vi "DblMonoPMDCurrentScan.vi"() -> ()   [LabVIEW 2010]
uses:
  <vilib>/DAQmx/write.llb/DAQmx Write (Analog DBL 1Chan 1Samp).vi
  <vilib>/DAQmx/read.llb/DAQmx Read (Analog 1D DBL 1Chan NSamp).vi
  <vilib>/DAQmx/create/channels.llb/DAQmx Create Channel (AO-Voltage-Basic).vi
  <vilib>/DAQmx/create/channels.llb/DAQmx Create Channel (AI-Voltage-Basic).vi
  <vilib>/daqmx/miscellaneous.llb/DAQmx Fill In Error Info.vi
  <vilib>/DAQmx/configure/timing.llb/DAQmx Timing (Sample Clock).vi
  <vilib>/Utility/file.llb/Write To Spreadsheet File (DBL).vi
  <vilib>/Analysis/NI_AALBase.lvlib
panel:
  in  "Voltage B":dbl min=-10.0 max=10.0 step=0.1 format="%0.2f"
  in  "Voltage A":dbl min=-10.0 max=10.0 step=0.1 format="%0.2f"
  in  "Output B":tag="Dev1/ao3"
  in  "Output A":tag="Dev1/ao2"
  in  "Input Channel":tag="Dev1/ai6"
  in  "Current":bool
  in  "Power":bool=TRUE
  out "ScanGraph":cluster{dbl[], dbl[]}(graph)
  in  "Sensitivity":dbl=1e-09 caption="(A/V)" format="%#_6p"
  out "Readout":dbl=-2.45576047e-07 format="%^#_9e"
  in  "Scan Save Path":path
  in  "On":bool=TRUE
  out "Waveform Chart":dbl(graph)=-2.45576047e-07
  in  "Save":bool=TRUE
  in  "Exit":bool
  in  "STOP":bool
  in  "Step Time (sec)":dbl=1.0 min=0.001 max=300.0 step=0.001 format="%.3f"
  in  "Step Size (nm)":dbl=1.0 min=0.1 max=100.0 step=0.1 format="%.1f"
  in  "End":dbl=800.0 min=0.0 max=2000.0 step=0.1 format="%.1f"
  in  "Start":dbl=400.0 min=0.0 max=2000.0 step=0.1 format="%.1f"
  in  "Scan":bool
  in  "Up":bool=TRUE caption="Down"
  in  "Increment (nm)":dbl=10.0 min=0.1 max=2000.0 step=0.1 format="%.1f"
  in  "PMD Settings":T1={"Beam Diameter (mm)"=4.0, "BWIn"=0, "Averaging Rate"=300, "Auto Range"=TRUE} {"Averaging Rate" min=33 max=5000 step=1; "BWIn" items=["HIGH", "LOW"]; "Beam Diameter (mm)" min=1.0 max=9.0 step=0.5}
  in  "Step":bool
  out "Busy":bool=TRUE
  in  "Send Command":bool
  in  "Command":u16(ring)=1 items=["nm", "goto", "nm/min", "VIS grating", "IR grating"]
  in  "Wavelength (nm)":dbl=500.0 min=0.0 max=2000.0 step=0.1 format="%.1f"
  in  "Scan Speed (nm/min)":dbl=100.0 min=1.0 max=500.0 step=0.1 format="%.1f"
  out "Done?":string="   ..."
  in  "Send Question":bool
  in  "Ask?":u16(ring) items=["?nm", "?nm/min", "?grating", "?turret", "?gratings"]
  in  "Zero?":bool
  out "PM Error log":string="-222,\"Data out of range\"\n-222,\"Data out of range\"\n-222,\"Data out of range\"\n-222,\"Data out of range\"\n-222,\"Data out of range\"\n-222,\"Data out of range\"\n-222,\"Data out of range\"\n-222,\"Data out of range\"\n-222,\"Data out of range\"\n-222,\"Data out of range\"\n-222,\"Data out of range\"\n-222,\"Data out of range\"\n-222,\"Data out of range\"\n-222,\"Data out of range\"\n-222,\"Data out of range\"\n-222,\"Data out of range\"\n-222,\"Data out of range\"\n-222,\"Data out of range\"\n-222,\"Data out of range\"\n-222,\"Data out of range\"\n-222,\"Data out of range\"\n-222,\"Data out of range\"\n-222,\"Data out of range\"\n-222,\"Data out of range\"\n-222,\"Data out of range\"\n-222,\"Data out of range\"\n-222,\"Data out of range\"\n-222,\"Data out of range\"\n-222,\"Data out of range\"\n-222,\"Data out of range\"\n-222,\"Data out of range\"\n-222,\"Data out of range\"\n-222,\"Data out of range\"\n-222,\"Data out of range\"\n-222,\"Data out of range\"\n-222,\"Data out of range\"\n-222,\"Data out of range\"\n-222,\"Data out of range\"\n-222,\"Data out of range\"\n-222,\"Data out of range\"\n-222,\"Data out of range\"\n-222,\"Data out of range\"\n-222,\"Data out of range\"\n-222,\"Data out of range\"\n-222,\"Data out of range\"\n-222,\"Data out of range\"\n-222,\"Data out of range\"\n-222,\"Data out of range\"\n-222,\"Data out of range\"\n-222,\"Data out of range\"\n-222,\"Data out of range\"\n-222,\"Data out of range\"\n-222,\"Data out of range\"\n-222,\"Data out of range\"\n-222,\"Data out of range\"\n-222,\"Data out of range\"\n-222,\"Data out of range\"\n-222,\"Data out of range\"\n-222,\"Data out of range\"\n-222,\"Data out of range\"\n-222,\"Data out of range\"\n-222,\"Data out of range\"\n-222,\"Data out of range\"\n-222,\"Data out of range\"\n-222,\"Data out of range\"\n-222,\"Data out of range\"\n-222,\"Data out of range\"\n-222,\"Data out of range\"\n-222,\"Data out of range\"\n-222,\"Data out of range\"\n-222,\"Data out of range\"\n-222,\"Data out of range\"\n-222,\"Data out of range\"\n-222,\"Data out of range\"\n-222,\"Data out of range\"\n-222,\"Data out of range\"\n-222,\"Data out of range\"\n-222,\"Data out of range\"\n-222,\"Data out of range\"\n-222,\"Data out of range\"\n-222,\"Data out of range\"\n-222,\"Data out of range\"\n-222,\"Data out of range\"\n-222,\"Data out of range\"\n-222,\"Data out of range\"\n-222,\"Data out of range\"\n-222,\"Data out of range\"\n-222,\"Data out of range\"\n-222,\"Data out of range\"\n-222,\"Data out of range\"\n-222,\"Data out of range\"\n-222,\"Data out of range\"\n-222,\"Data out of range\"\n-222,\"Data out of range\"\n-222,\"Data out of range\"\n-222,\"Data out of range\"\n-222,\"Data out of range\"\n-222,\"Data out of range\"\n-222,\"Data out of range\"\n-222,\"Data out of range\"\n-222,\"Data out of range\"\n-222,\"Data out of range\"\n-222,\"Data out of range\"\n-222,\"Data out of range\"\n-222,\"Data out of range\"\n-222,\"Data out of range\"\n-222,\"Data out of range\"\n-222,\"Data out of range\"\n-222,\"Data out of range\"\n-222,\"Data out of range\"\n-222,\"Data out of range\"\n-222,\"Data out of range\"\n-222,\"Data out of range\"\n-222,\"Data out of range\"\n-222,\"Data out of range\"\n-222,\"Data out of range\"\n-222,\"Data out of range\"\n-222,\"Data out of range\"\n-222,\"Data out of range\"\n-222,\"Data out of range\"\n-222,\"Data out of range\"\n-222,\"Data out of range\"\n-222,\"Data out of range\"\n-222,\"Data out of range\"\n-222,\"Data out of range\"\n-222,\"Data out of range\"\n-222,\"Data out of range\"\n-222,\"Data out of range\"\n-222,\"Data out of range\"\n-222,\"Data out of range\"\n-222,\"Data out of range\"\n-222,\"Data out of range\"\n-222,\"Data out of range\"\n-222,\"Data out of range\"\n-222,\"Data out of range\"\n-222,\"Data out of range\"\n-222,\"Data out of range\"\n-222,\"Data out of range\"\n-222,\"Data out of range\"\n-222,\"Data out of range\"\n-222,\"Data out of range\"\n-222,\"Data out of range\"\n-222,\"Data out of range\"\n-222,\"Data out of range\"\n-222,\"Data out of range\"\n-222,\"Data out of range\"\n-222,\"Data out of range\"\n-222,\"Data out of range\"\n-222,\"Data out of range\"\n-222,\"Data out of range\"\n-222,\"Data out of range\"\n-222,\"Data out of range\"\n-222,\"Data out of range\"\n-222,\"Data out of range\"\n-222,\"Data out of range\"\n-222,\"Data out of range\"\n-222,\"Data out of range\"\n-222,\"Data out of range\"\n-222,\"Data out of range\"\n-222,\"Data out of range\"\n-222,\"Data out of range\"\n-222,\"Data out of range\"\n-222,\"Data out of range\"\n-222,\"Data out of range\"\n-222,\"Data out of range\"\n-222,\"Data out of range\"\n-222,\"Data out of range\"\n-222,\"Data out of range\"\n-222,\"Data out of range\"\n-222,\"Data out of range\"\n-222,\"Data out of range\"\n-222,\"Data out of range\"\n-222,\"Data out of range\"\n-222,\"Data out of range\"\n-222,\"Data out of range\"\n-222,\"Data out of range\"\n-222,\"Data out of range\"\n-222,\"Data out of range\"\n-222,\"Data out of range\"\n-222,\"Data out of range\"\n-222,\"Data out of range\"\n-222,\"Data out of range\"\n-222,\"Data out of range\"\n-222,\"Data out of range\"\n-222,\"Data out of range\"\n-222,\"Data out of range\"\n-222,\"Data out of range\"\n-222,\"Data out of range\"\n-222,\"Data out of range\"\n-222,\"Data out of range\"\n-222,\"Data out of range\"\n-222,\"Data out of range\"\n-222,\"Data out of range\"\n-222,\"Data out of range\"\n-222,\"Data out of range\"\n-222,\"Data out of range\"\n-222,\"Data out of range\"\n-222,\"Data out of range\"\n-222,\"Data out of range\"\n-222,\"Data out of range\"\n-222,\"Data out of range\"\n-222,\"Data out of range\"\n-222,\"Data out of range\"\n-222,\"Data out of range\"\n-222,\"Data out of range\"\n-222,\"Data out of range\"\n-222,\"Data out of range\"\n-222,\"Data out of range\"\n-222,\"Data out of range\"\n-222,\"Data out of range\"\n-222,\"Data out of range\"\n-222,\"Data out of range\"\n-222,\"Data out of range\"\n-222,\"Data out of range\"\n-222,\"Data out of range\"\n-222,\"Data out of range\"\n-222,\"Data out of range\"\n-222,\"Data out of range\"\n-222,\"Data out of range\"\n-222,\"Data out of range\"\n-222,\"Data out of range\"\n-222,\"Data out of range\"\n-222,\"Data out of range\"\n-222,\"Data out of range\"\n-222,\"Data out of range\"\n-222,\"Data out of range\"\n-222,\"Data out of range\"\n-222,\"Data out of range\"\n-222,\"Data out of range\"\n-222,\"Data out of range\"\n-222,\"Data out of range\"\n-222,\"Data out of range\"\n-222,\"Data out of range\"\n-222,\"Data out of range\"\n-222,\"Data out of range\"\n-222,\"Data out of range\"\n-222,\"Data out of range\"\n-222,\"Data out of range\"\n-222,\"Data out of range\"\n-222,\"Data out of range\"\n-222,\"Data out of range\"\n-222,\"Data out of range\"\n-222,\"Data out of range\"\n-222,\"Data out of range\"\n-222,\"Data out of range\"\n-222,\"Data out of range\"\n-222,\"Data out of range\"\n-222,\"Data out of range\"\n-222,\"Data out of range\"\n-222,\"Data out of range\"\n-222,\"Data out of range\"\n-222,\"Data out of range\"\n-222,\"Data out of range\"\n-222,\"Data out of range\"\n-222,\"Data out of range\"\n-222,\"Data out of range\"\n-222,\"Data out of range\"\n-222,\"Data out of range\"\n-222,\"Data out of range\"\n-222,\"Data out of range\"\n-222,\"Data out of range\"\n-222,\"Data out of range\"\n-222,\"Data out of range\"\n-222,\"Data out of range\"\n-222,\"Data out of range\"\n-222,\"Data out of range\"\n-222,\"Data out of range\"\n-222,\"Data out of range\"\n-222,\"Data out of range\"\n-222,\"Data out of range\"\n-222,\"Data out of range\"\n-222,\"Data out of range\"\n-222,\"Data out of range\"\n-222,\"Data out of range\"\n-222,\"Data out of range\"\n-222,\"Data out of range\"\n-222,\"Data out of range\"\n-222,\"Data out of range\"\n-222,\"Data out of range\"\n-222,\"Data out of range\"\n-222,\"Data out of range\"\n-222,\"Data out of range\"\n-222,\"Data out of range\"\n-222,\"Data out of range\"\n-222,\"Data out of range\"\n-222,\"Data out of range\"\n-222,\"Data out of range\"\n-222,\"Data out of range\"\n-222,\"Data out of range\"\n-222,\"Data out of range\"\n-222,\"Data out of range\"\n-222,\"Data out of range\"\n-222,\"Data out of range\"\n-222,\"Data out of range\"\n-222,\"Data out of range\"\n-222,\"Data out of range\"\n-222,\"Data out of range\"\n-222,\"Data out of range\"\n-222,\"Data out of range\"\n-222,\"Data out of range\"\n-222,\"Data out of range\"\n-222,\"Data out of range\"\n-222,\"Data out of range\"\n-222,\"Data out of range\"\n-222,\"Data out of range\"\n-222,\"Data out of range\"\n-222,\"Data out of range\"\n-222,\"Data out of range\"\n-222,\"Data out of range\"\n-222,\"Data out of range\"\n-222,\"Data out of range\"\n-222,\"Data out of range\"\n-222,\"Data out of range\"\n-222,\"Data out of range\"\n-222,\"Data out of range\"\n-222,\"Data out of range\"\n-222,\"Data out of range\"\n-222,\"Data out of range\"\n-222,\"Data out of range\"\n-222,\"Data out of range\"\n-222,\"Data out of range\"\n-222,\"Data out of range\"\n-222,\"Data out of range\"\n-222,\"Data out of range\"\n-222,\"Data out of range\"\n-222,\"Data out of range\"\n-222,\"Data out of range\"\n-222,\"Data out of range\"\n-222,\"Data out of range\"\n-222,\"Data out of range\"\n-222,\"Data out of range\"\n-222,\"Data out of range\"\n-222,\"Data out of range\"\n-222,\"Data out of range\"\n-222,\"Data out of range\"\n-222,\"Data out of range\"\n-222,\"Data out of range\"\n-222,\"Data out of range\"\n-222,\"Data out of range\"\n-222,\"Data out of range\"\n-222,\"Data out of range\"\n-222,\"Data out of range\"\n-222,\"Data out of range\"\n-222,\"Data out of range\"\n-222,\"Data out of range\"\n-222,\"Data out of range\"\n-222,\"Data out of range\"\n-222,\"Data out of range\"\n-222,\"Data out of range\"\n-222,\"Data out of range\"\n-222,\"Data out of range\"\n-222,\"Data out of range\"\n-222,\"Data out of range\"\n-222,\"Data out of range\"\n-222,\"Data out of range\"\n-222,\"Data out of range\"\n-222,\"Data out of range\"\n-222,\"Data out of range\"\n-222,\"Data out of range\"\n-222,\"Data out of range\"\n-222,\"Data out of range\"\n-222,\"Data out of range\"\n-222,\"Data out of range\"\n-222,\"Data out of range\"\n-222,\"Data out of range\"\n-222,\"Data out of range\"\n-222,\"Data out of range\"\n-222,\"Data out of range\"\n-222,\"Data out of range\"\n-222,\"Data out of range\"\n-222,\"Data out of range\"\n-222,\"Data out of range\"\n-222,\"Data out of range\"\n-222,\"Data out of range\"\n-222,\"Data out of range\"\n-222,\"Data out of range\"\n-222,\"Data out of range\"\n-222,\"Data out of range\"\n-222,\"Data out of range\"\n-222,\"Data out of range\"\n-222,\"Data out of range\"\n-222,\"Data out of range\"\n-222,\"Data out of range\"\n-222,\"Data out of range\"\n-222,\"Data out of range\"\n-222,\"Data out of range\"\n-222,\"Data out of range\"\n-222,\"Data out of range\"\n-222,\"Data out of range\"\n-222,\"Data out of range\"\n-222,\"Data out of range\"\n-222,\"Data out of range\"\n-222,\"Data out of range\"\n-222,\"Data out of range\"\n-222,\"Data out of range\"\n-222,\"Data out of range\"\n-222,\"Data out of range\"\n-222,\"Data out of range\"\n-222,\"Data out of range\"\n-222,\"Data out of range\"\n-222,\"Data out of range\"\n-222,\"Data out of range\"\n-222,\"Data out of range\"\n-222,\"Data out of range\"\n-222,\"Data out of range\"\n-222,\"Data out of range\"\n-222,\"Data out of range\"\n-222,\"Data out of range\"\n-222,\"Data out of range\"\n-222,\"Data out of range\"\n-222,\"Data out of range\"\n-222,\"Data out of range\"\n-222,\"Data out of range\"\n-222,\"Data out of range\"\n-222,\"Data out of range\"\n-222,\"Data out of range\"\n-222,\"Data out of range\"\n-222,\"Data out of range\"\n-222,\"Data out of range\"\n-222,\"Data out of range\"\n-222,\"Data out of range\"\n-222,\"Data out of range\"\n-222,\"Data out of range\"\n-222,\"Data out of range\"\n-222,\"Data out of range\"\n-222,\"Data out of range\"\n-222,\"Data out of range\"\n-222,\"Data out of range\"\n-222,\"Data out of range\"\n-222,\"Data out of range\"\n-222,\"Data out of range\"\n-222,\"Data out of range\"\n-222,\"Data out of range\"\n-222,\"Data out of range\"\n-222,\"Data out of range\"\n-222,\"Data out of range\"\n-222,\"Data out of range\"\n-222,\"Data out of range\"\n-222,\"Data out of range\"\n-222,\"Data out of range\"\n-222,\"Data out of range\"\n-222,\"Data out of range\"\n-222,\"Data out of range\"\n-222,\"Data out of range\"\n-222,\"Data out of range\"\n-222,\"Data out of range\"\n-222,\"Data out of range\"\n-222,\"Data out of range\"\n-222,\"Data out of range\"\n-222,\"Data out of range\"\n-222,\"Data out of range\"\n-222,\"Data out of range\"\n-222,\"Data out of range\"\n-222,\"Data out of range\"\n-222,\"Data out of range\"\n-222,\"Data out of range\"\n-222,\"Data out of range\"\n-222,\"Data out of range\"\n-222,\"Data out of range\"\n-222,\"Data out of range\"\n-222,\"Data out of range\"\n-222,\"Data out of range\"\n-222,\"Data out of range\"\n-222,\"Data out of range\"\n-222,\"Data out of range\"\n-222,\"Data out of range\"\n-222,\"Data out of range\"\n-222,\"Data out of range\"\n-222,\"Data out of range\"\n-222,\"Data out of range\"\n-222,\"Data out of range\"\n-222,\"Data out of range\"\n-222,\"Data out of range\"\n-222,\"Data out of range\"\n-222,\"Data out of range\"\n-222,\"Data out of range\"\n-222,\"Data out of range\"\n-222,\"Data out of range\"\n-222,\"Data out of range\"\n-222,\"Data out of range\"\n-222,\"Data out of range\"\n-222,\"Data out of range\"\n-222,\"Data out of range\"\n-222,\"Data out of range\"\n-222,\"Data out of range\"\n-222,\"Data out of range\"\n-222,\"Data out of range\"\n-222,\"Data out of range\"\n-222,\"Data out of range\"\n-222,\"Data out of range\"\n-222,\"Data out of range\"\n-222,\"Data out of range\"\n-222,\"Data out of range\"\n-222,\"Data out of range\"\n-222,\"Data out of range\"\n-222,\"Data out of range\"\n-222,\"Data out of range\"\n-222,\"Data out of range\"\n-222,\"Data out of range\"\n-222,\"Data out of range\"\n-222,\"Data out of range\"\n-222,\"Data out of range\"\n-222,\"Data out of range\"\n-222,\"Data out of range\"\n-222,\"Data out of range\"\n-222,\"Data out of range\"\n-222,\"Data out of range\"\n-222,\"Data out of range\"\n-222,\"Data out of range\"\n-222,\"Data out of range\"\n-222,\"Data out of range\"\n-222,\"Data out of range\"\n-222,\"Data out of range\"\n-222,\"Data out of range\"\n-222,\"Data out of range\"\n-222,\"Data out of range\"\n-222,\"Data out of range\"\n-222,\"Data out of range\"\n-222,\"Data out of range\"\n-222,\"Data out of range\"\n-222,\"Data out of range\"\n-222,\"Data out of range\"\n-222,\"Data out of range\"\n-222,\"Data out of range\"\n-222,\"Data out of range\"\n-222,\"Data out of range\"\n-222,\"Data out of range\"\n-222,\"Data out of range\"\n-222,\"Data out of range\"\n-222,\"Data out of range\"\n-222,\"Data out of range\"\n-222,\"Data out of range\"\n-222,\"Data out of range\"\n-222,\"Data out of range\"\n-222,\"Data out of range\"\n-222,\"Data out of range\"\n-222,\"Data out of range\"\n-222,\"Data out of range\"\n-222,\"Data out of range\"\n-222,\"Data out of range\"\n-222,\"Data out of range\"\n-222,\"Data out of range\"\n-222,\"Data out of range\"\n-222,\"Data out of range\"\n-222,\"Data out of range\"\n-222,\"Data out of range\"\n-222,\"Data out of range\"\n-222,\"Data out of range\"\n-222,\"Data out of range\"\n-222,\"Data out of range\"\n-222,\"Data out of range\"\n-222,\"Data out of range\"\n-222,\"Data out of range\"\n-222,\"Data out of range\"\n-222,\"Data out of range\"\n-222,\"Data out of range\"\n-222,\"Data out of range\"\n-222,\"Data out of range\"\n-222,\"Data out of range\"\n-222,\"Data out of range\"\n-222,\"Data out of range\"\n-222,\"Data out of range\"\n-222,\"Data out of range\"\n-222,\"Data out of range\"\n-222,\"Data out of range\"\n-222,\"Data out of range\"\n-222,\"Data out of range\"\n-222,\"Data out of range\"\n-222,\"Data out of range\"\n-222,\"Data out of range\"\n-222,\"Data out of range\"\n-222,\"Data out of range\"\n-222,\"Data out of range\"\n-222,\"Data out of range\"\n-222,\"Data out of range\"\n-222,\"Data out of range\"\n-222,\"Data out of range\"\n-222,\"Data out of range\"\n-222,\"Data out of range\"\n-222,\"Data out of range\"\n-222,\"Data out of range\"\n-222,\"Data out of range\"\n-222,\"Data out of range\"\n-222,\"Data out of range\"\n-222,\"Data out of range\"\n-222,\"Data out of range\"\n-222,\"Data out of range\"\n-222,\"Data out of range\"\n-222,\"Data out of range\"\n-222,\"Data out of range\"\n-222,\"Data out of range\"\n-222,\"Data out of range\"\n-222,\"Data out of range\"\n-222,\"Data out of range\"\n-222,\"Data out of range\"\n-222,\"Data out of range\"\n-222,\"Data out of range\"\n-222,\"Data out of range\"\n-222,\"Data out of range\"\n-222,\"Data out of range\"\n-222,\"Data out of range\"\n-222,\"Data out of range\"\n-222,\"Data out of range\"\n-222,\"Data out of range\"\n-222,\"Data out of range\"\n-222,\"Data out of range\"\n-222,\"Data out of range\"\n-222,\"Data out of range\"\n-222,\"Data out of range\"\n-222,\"Data out of range\"\n-222,\"Data out of range\"\n-222,\"Data out of range\"\n-222,\"Data out of range\"\n-222,\"Data out of range\"\n-222,\"Data out of range\"\n-222,\"Data out of range\"\n-222,\"Data out of range\"\n-222,\"Data out of range\"\n-222,\"Data out of range\"\n-222,\"Data out of range\"\n-222,\"Data out of range\"\n-222,\"Data out of range\"\n-222,\"Data out of range\"\n-222,\"Data out of range\"\n-222,\"Data out of range\"\n-222,\"Data out of range\"\n-222,\"Data out of range\"\n-222,\"Data out of range\"\n-222,\"Data out of range\"\n-222,\"Data out of range\"\n-222,\"Data out of range\"\n-222,\"Data out of range\"\n-222,\"Data out of range\"\n-222,\"Data out of range\"\n-222,\"Data out of range\"\n-222,\"Data out of range\"\n-222,\"Data out of range\"\n-222,\"Data out of range\"\n-222,\"Data out of range\"\n-222,\"Data out of range\"\n-222,\"Data out of range\"\n-222,\"Data out of range\"\n-222,\"Data out of range\"\n-222,\"Data out of range\"\n-222,\"Data out of range\"\n-222,\"Data out of range\"\n-222,\"Data out of range\"\n-222,\"Data out of range\"\n-222,\"Data out of range\"\n-222,\"Data out of range\"\n-222,\"Data out of range\"\n-222,\"Data out of range\"\n-222,\"Data out of range\"\n-222,\"Data out of range\"\n-222,\"Data out of range\"\n-222,\"Data out of range\"\n-222,\"Data out of range\"\n-222,\"Data out of range\"\n-222,\"Data out of range\"\n-222,\"Data out of range\"\n-222,\"Data out of range\"\n-222,\"Data out of range\"\n-222,\"Data out of range\"\n-222,\"Data out of range\"\n-222,\"Data out of range\"\n-222,\"Data out of range\"\n-222,\"Data out of range\"\n-222,\"Data out of range\"\n-222,\"Data out of range\"\n-222,\"Data out of range\"\n-222,\"Data out of range\"\n-222,\"Data out of range\"\n-222,\"Data out of range\"\n-222,\"Data out of range\"\n-222,\"Data out of range\"\n-222,\"Data out of range\"\n-222,\"Data out of range\"\n-222,\"Data out of range\"\n-222,\"Data out of range\"\n-222,\"Data out of range\"\n-222,\"Data out of range\"\n-222,\"Data out of range\"\n-222,\"Data out of range\"\n-222,\"Data out of range\"\n-222,\"Data out of range\"\n-222,\"Data out of range\"\n-222,\"Data out of range\"\n-222,\"Data out of range\"\n-222,\"Data out of range\"\n-222,\"Data out of range\"\n-222,\"Data out of range\"\n-222,\"Data out of range\"\n-222,\"Data out of range\"\n-222,\"Data out of range\"\n-222,\"Data out of range\"\n-222,\"Data out of range\"\n-222,\"Data out of range\"\n-222,\"Data out of range\"\n-222,\"Data out of range\"\n-222,\"Data out of range\"\n-222,\"Data out of range\"\n-222,\"Data out of range\"\n-222,\"Data out of range\"\n-222,\"Data out of range\"\n-222,\"Data out of range\"\n-222,\"Data out of range\"\n-222,\"Data out of range\"\n-222,\"Data out of range\"\n-222,\"Data out of range\"\n-222,\"Data out of range\"\n-222,\"Data out of range\"\n-222,\"Data out of range\"\n-222,\"Data out of range\"\n-222,\"Data out of range\"\n-222,\"Data out of range\"\n-222,\"Data out of range\"\n-222,\"Data out of range\"\n-222,\"Data out of range\"\n-222,\"Data out of range\"\n-222,\"Data out of range\"\n-222,\"Data out of range\"\n-222,\"Data out of range\"\n-222,\"Data out of range\"\n-222,\"Data out of range\"\n-222,\"Data out of range\"\n-222,\"Data out of range\"\n-222,\"Data out of range\"\n-222,\"Data out of range\"\n-222,\"Data out of range\"\n-222,\"Data out of range\"\n-222,\"Data out of range\"\n-222,\"Data out of range\"\n-222,\"Data out of range\"\n-222,\"Data out of range\"\n-222,\"Data out of range\"\n-222,\"Data out of range\"\n-222,\"Data out of range\"\n-222,\"Data out of range\"\n-222,\"Data out of range\"\n-222,\"Data out of range\"\n-222,\"Data out of range\"\n-222,\"Data out of range\"\n-222,\"Data out of range\"\n-222,\"Data out of range\"\n-222,\"Data out of range\"\n-222,\"Data out of range\"\n-222,\"Data out of range\"\n-222,\"Data out of range\"\n-222,\"Data out of range\"\n-222,\"Data out of range\"\n-222,\"Data out of range\"\n-222,\"Data out of range\"\n-222,\"Data out of range\"\n-222,\"Data out of range\"\n-222,\"Data out of range\"\n-222,\"Data out of range\"\n-222,\"Data out of range\"\n-222,\"Data out of range\"\n-222,\"Data out of range\"\n-222,\"Data out of range\"\n-222,\"Data out of range\"\n-222,\"Data out of range\"\n-222,\"Data out of range\"\n-222,\"Data out of range\"\n-222,\"Data out of range\"\n-222,\"Data out of range\"\n-222,\"Data out of range\"\n-222,\"Data out of range\"\n-222,\"Data out of range\"\n-222,\"Data out of range\"\n-222,\"Data out of range\"\n-222,\"Data out of range\"\n-222,\"Data out of range\"\n-222,\"Data out of range\"\n-222,\"Data out of range\"\n-222,\"Data out of range\"\n-222,\"Data out of range\"\n-222,\"Data out of range\"\n-222,\"Data out of range\"\n-222,\"Data out of range\"\n-222,\"Data out of range\"\n-222,\"Data out of range\"\n-222,\"Data out of range\"\n-222,\"Data out of range\"\n-222,\"Data out of range\"\n-222,\"Data out of range\"\n-222,\"Data out of range\"\n-222,\"Data out of range\"\n-222,\"Data out of range\"\n-222,\"Data out of range\"\n-222,\"Data out of range\"\n-222,\"Data out of range\"\n-222,\"Data out of range\"\n-222,\"Data out of range\"\n-222,\"Data out of range\"\n-222,\"Data out of range\"\n-222,\"Data out of range\"\n-222,\"Data out of range\"\n-222,\"Data out of range\"\n-222,\"Data out of range\"\n-222,\"Data out of range\"\n-222,\"Data out of range\"\n-222,\"Data out of range\"\n-222,\"Data out of range\"\n-222,\"Data out of range\"\n-222,\"Data out of range\"\n-222,\"Data out of range\"\n-222,\"Data out of range\"\n-222,\"Data out of range\"\n-222,\"Data out of range\"\n-222,\"Data out of range\"\n-222,\"Data out of range\"\n-222,\"Data out of range\"\n-222,\"Data out of range\"\n-222,\"Data out of range\"\n-222,\"Data out of range\"\n-222,\"Data out of range\"\n-222,\"Data out of range\"\n-222,\"Data out of range\"\n-222,\"Data out of range\"\n-222,\"Data out of range\"\n-222,\"Data out of range\"\n-222,\"Data out of range\"\n-222,\"Data out of range\"\n-222,\"Data out of range\"\n-222,\"Data out of range\"\n-222,\"Data out of range\"\n-222,\"Data out of range\"\n-222,\"Data out of range\"\n-222,\"Data out of range\"\n-222,\"Data out of range\"\n-222,\"Data out of range\"\n-222,\"Data out of range\"\n-222,\"Data out of range\"\n-222,\"Data out of range\"\n-222,\"Data out of range\"\n-222,\"Data out of range\"\n-222,\"Data out of range\"\n-222,\"Data out of range\"\n-222,\"Data out of range\"\n-222,\"Data out of range\"\n-222,\"Data out of range\"\n-222,\"Data out of range\"\n-222,\"Data out of range\"\n-222,\"Data out of range\"\n-222,\"Data out of range\"\n-222,\"Data out of range\"\n-222,\"Data out of range\"\n-222,\"Data out of range\"\n-222,\"Data out of range\"\n-222,\"Data out of range\"\n-222,\"Data out of range\"\n-222,\"Data out of range\"\n-222,\"Data out of range\"\n-222,\"Data out of range\"\n-222,\"Data out of range\"\n-222,\"Data out of range\"\n-222,\"Data out of range\"\n-222,\"Data out of range\"\n-222,\"Data out of range\"\n-222,\"Data out of range\"\n-222,\"Data out of range\"\n-222,\"Data out of range\"\n-222,\"Data out of range\"\n-222,\"Data out of range\"\n-222,\"Data out of range\"\n-222,\"Data out of range\"\n-222,\"Data out of range\"\n-222,\"Data out of range\"\n-222,\"Data out of range\"\n-222,\"Data out of range\"\n-222,\"Data out of range\"\n-222,\"Data out of range\"\n-222,\"Data out of range\"\n-222,\"Data out of range\"\n-222,\"Data out of range\"\n-222,\"Data out of range\"\n-222,\"Data out of range\"\n-222,\"Data out of range\"\n-222,\"Data out of range\"\n-222,\"Data out of range\"\n-222,\"Data out of range\"\n-222,\"Data out of range\"\n-222,\"Data out of range\"\n-222,\"Data out of range\"\n-222,\"Data out of range\"\n-222,\"Data out of range\"\n-222,\"Data out of range\"\n-222,\"Data out of range\"\n-222,\"Data out of range\"\n-222,\"Data out of range\"\n-222,\"Data out of range\"\n-222,\"Data out of range\"\n-222,\"Data out of range\"\n-222,\"Data out of range\"\n-222,\"Data out of range\"\n-222,\"Data out of range\"\n-222,\"Data out of range\"\n-222,\"Data out of range\"\n-222,\"Data out of range\"\n-222,\"Data out of range\"\n-222,\"Data out of range\"\n-222,\"Data out of range\"\n-222,\"Data out of range\"\n-222,\"Data out of range\"\n-222,\"Data out of range\"\n-222,\"Data out of range\"\n-222,\"Data out of range\"\n-222,\"Data out of range\"\n-222,\"Data out of range\"\n-222,\"Data out of range\"\n-222,\"Data out of range\"\n-222,\"Data out of range\"\n-222,\"Data out of range\"\n-222,\"Data out of range\"\n-222,\"Data out of range\"\n-222,\"Data out of range\"\n-222,\"Data out of range\"\n-222,\"Data out of range\"\n-222,\"Data out of range\"\n-222,\"Data out of range\"\n-222,\"Data out of range\"\n-222,\"Data out of range\"\n-222,\"Data out of range\"\n-222,\"Data out of range\"\n-222,\"Data out of range\"\n-222,\"Data out of range\"\n-222,\"Data out of range\"\n-222,\"Data out of range\"\n-222,\"Data out of range\"\n-222,\"Data out of range\"\n-222,\"Data out of range\"\n-222,\"Data out of range\"\n-222,\"Data out of range\"\n-222,\"Data out of range\"\n-222,\"Data out of range\"\n-222,\"Data out of range\"\n-222,\"Data out of range\"\n-222,\"Data out of range\"\n-222,\"Data out of range\"\n-222,\"Data out of range\"\n-222,\"Data out of range\"\n-222,\"Data out of range\"\n-222,\"Data out of range\"\n-222,\"Data out of range\"\n-222,\"Data out of range\"\n-222,\"Data out of range\"\n-222,\"Data out of range\"\n-222,\"Data out of range\"\n-222,\"Data out of range\"\n-222,\"Data out of range\"\n-222,\"Data out of range\"\n-222,\"Data out of range\"\n-222,\"Data out of range\"\n-222,\"Data out of range\"\n-222,\"Data out of range\"\n-222,\"Data out of range\"\n-222,\"Data out of range\"\n-222,\"Data out of range\"\n-222,\"Data out of range\"\n-222,\"Data out of range\"\n-222,\"Data out of range\"\n-222,\"Data out of range\"\n-222,\"Data out of range\"\n-222,\"Data out of range\"\n-222,\"Data out of range\"\n-222,\"Data out of range\"\n-222,\"Data out of range\"\n-222,\"Data out of range\"\n-222,\"Data out of range\"\n-222,\"Data out of range\"\n-222,\"Data out of range\"\n-222,\"Data out of range\"\n-222,\"Data out of range\"\n-222,\"Data out of range\"\n-222,\"Data out of range\"\n-222,\"Data out of range\"\n-222,\"Data out of range\"\n-222,\"Data out of range\"\n-222,\"Data out of range\"\n-222,\"Data out of range\"\n-222,\"Data out of range\"\n-222,\"Data out of range\"\n-222,\"Data out of range\"\n-222,\"Data out of range\"\n-222,\"Data out of range\"\n-222,\"Data out of range\"\n-222,\"Data out of range\"\n-222,\"Data out of range\"\n-222,\"Data out of range\"\n-222,\"Data out of range\"\n-222,\"Data out of range\"\n-222,\"Data out of range\"\n-222,\"Data out of range\"\n-222,\"Data out of range\"\n-222,\"Data out of range\"\n-222,\"Data out of range\"\n-222,\"Data out of range\"\n-222,\"Data out of range\"\n-222,\"Data out of range\"\n-222,\"Data out of range\"\n-222,\"Data out of range\"\n-222,\"Data out of range\"\n-222,\"Data out of range\"\n-222,\"Data out of range\"\n-222,\"Data out of range\"\n-222,\"Data out of range\"\n-222,\"Data out of range\"\n-222,\"Data out of range\"\n-222,\"Data out of range\"\n-222,\"Data out of range\"\n-222,\"Data out of range\"\n-222,\"Data out of range\"\n-222,\"Data out of range\"\n-222,\"Data out of range\"\n-222,\"Data out of range\"\n-222,\"Data out of range\"\n-222,\"Data out of range\"\n-222,\"Data out of range\"\n-222,\"Data out of range\"\n-222,\"Data out of range\"\n-222,\"Data out of range\"\n-222,\"Data out of range\"\n-222,\"Data out of range\"\n-222,\"Data out of range\"\n-222,\"Data out of range\"\n-222,\"Data out of range\"\n-222,\"Data out of range\"\n-222,\"Data out of range\"\n-222,\"Data out of range\"\n-222,\"Data out of range\"\n-222,\"Data out of range\"\n-222,\"Data out of range\"\n-222,\"Data out of range\"\n-222,\"Data out of range\"\n-222,\"Data out of range\"\n-222,\"Data out of range\"\n-222,\"Data out of range\"\n-222,\"Data out of range\"\n-222,\"Data out of range\"\n-222,\"Data out of range\"\n-222,\"Data out of range\"\n-222,\"Data out of range\"\n-222,\"Data out of range\"\n-222,\"Data out of range\"\n-222,\"Data out of range\"\n-222,\"Data out of range\"\n-222,\"Data out of range\"\n-222,\"Data out of range\"\n-222,\"Data out of range\"\n-222,\"Data out of range\"\n-222,\"Data out of range\"\n-222,\"Data out of range\"\n-222,\"Data out of range\"\n-222,\"Data out of range\"\n-222,\"Data out of range\"\n-222,\"Data out of range\"\n-222,\"Data out of range\"\n-222,\"Data out of range\"\n-222,\"Data out of range\"\n-222,\"Data out of range\"\n-222,\"Data out of range\"\n-222,\"Data out of range\"\n-222,\"Data out of range\"\n-222,\"Data out of range\"\n-222,\"Data out of range\"\n-222,\"Data out of range\"\n-222,\"Data out of range\"\n-222,\"Data out of range\"\n-222,\"Data out of range\"\n-222,\"Data out of range\"\n-222,\"Data out of range\"\n-222,\"Data out of range\"\n-222,\"Data out of range\"\n-222,\"Data out of range\"\n-222,\"Data out of range\"\n-222,\"Data out of range\"\n-222,\"Data out of range\"\n-222,\"Data out of range\"\n-222,\"Data out of range\"\n-222,\"Data out of range\"\n-222,\"Data out of range\"\n-222,\"Data out of range\"\n-222,\"Data out of range\"\n-222,\"Data out of range\"\n-222,\"Data out of range\"\n-222,\"Data out of range\"\n-222,\"Data out of range\"\n-222,\"Data out of range\"\n-222,\"Data out of range\"\n-222,\"Data out of range\"\n-222,\"Data out of range\"\n-222,\"Data out of range\"\n-222,\"Data out of range\"\n-222,\"Data out of range\"\n-222,\"Data out of range\"\n-222,\"Data out of range\"\n-222,\"Data out of range\"\n-222,\"Data out of range\"\n-222,\"Data out of range\"\n-222,\"Data out of range\"\n-222,\"Data out of range\"\n-222,\"Data out of range\"\n-222,\"Data out of range\"\n-222,\"Data out of range\"\n-222,\"Data out of range\"\n-222,\"Data out of range\"\n-222,\"Data out of range\"\n-222,\"Data out of range\"\n-222,\"Data out of range\"\n-222,\"Data out of range\"\n-222,\"Data out of range\"\n-222,\"Data out of range\"\n-222,\"Data out of range\"\n-222,\"Data out of range\"\n-222,\"Data out of range\"\n-222,\"Data out of range\"\n-222,\"Data out of range\"\n-222,\"Data out of range\"\n-222,\"Data out of range\"\n-222,\"Data out of range\"\n-222,\"Data out of range\"\n-222,\"Data out of range\"\n-222,\"Data out of range\"\n-222,\"Data out of range\"\n-222,\"Data out of range\"\n-222,\"Data out of range\"\n-222,\"Data out of range\"\n-222,\"Data out of range\"\n-222,\"Data out of range\"\n-222,\"Data out of range\"\n-222,\"Data out of range\"\n-222,\"Data out of range\"\n-222,\"Data out of range\"\n-222,\"Data out of range\"\n-222,\"Data out of range\"\n-222,\"Data out of range\"\n-222,\"Data out of range\"\n-222,\"Data out of range\"\n-222,\"Data out of range\"\n-222,\"Data out of range\"\n-222,\"Data out of range\"\n-222,\"Data out of range\"\n-222,\"Data out of range\"\n-222,\"Data out of range\"\n-222,\"Data out of range\"\n-222,\"Data out of range\"\n-222,\"Data out of range\"\n-222,\"Data out of range\"\n-222,\"Data out of range\"\n-222,\"Data out of range\"\n-222,\"Data out of range\"\n-222,\"Data out of range\"\n-222,\"Data out of range\"\n-222,\"Data out of range\"\n-222,\"Data out of range\"\n-222,\"Data out of range\"\n-222,\"Data out of range\"\n-222,\"Data out of range\"\n-222,\"Data out of range\"\n-222,\"Data out of range\"\n-222,\"Data out of range\"\n-222,\"Data out of range\"\n-222,\"Data out of range\"\n-222,\"Data out of range\"\n-222,\"Data out of range\"\n-222,\"Data out of range\"\n-222,\"Data out of range\"\n-222,\"Data out of range\"\n-222,\"Data out of range\"\n-222,\"Data out of range\"\n-222,\"Data out of range\"\n-222,\"Data out of range\"\n-222,\"Data out of range\"\n-222,\"Data out of range\"\n-222,\"Data out of range\"\n-222,\"Data out of range\"\n-222,\"Data out of range\"\n-222,\"Data out of range\"\n-222,\"Data out of range\"\n-222,\"Data out of range\"\n-222,\"Data out of range\"\n-222,\"Data out of range\"\n-222,\"Data out of range\"\n-222,\"Data out of range\"\n-222,\"Data out of range\"\n-222,\"Data out of range\"\n-222,\"Data out of range\"\n-222,\"Data out of range\"\n-222,\"Data out of range\"\n-222,\"Data out of range\"\n-222,\"Data out of range\"\n-222,\"Data out of range\"\n-222,\"Data out of range\"\n-222,\"Data out of range\"\n-222,\"Data out of range\"\n-222,\"Data out of range\"\n-222,\"Data out of range\"\n-222,\"Data out of range\"\n-222,\"Data out of range\"\n-222,\"Data out of range\"\n-222,\"Data out of range\"\n-222,\"Data out of range\"\n-222,\"Data out of range\"\n-222,\"Data out of range\"\n-222,\"Data out of range\"\n-222,\"Data out of range\"\n-222,\"Data out of range\"\n-222,\"Data out of range\"\n-222,\"Data out of range\"\n-222,\"Data out of range\"\n-222,\"Data out of range\"\n-222,\"Data out of range\"\n-222,\"Data out of range\"\n-222,\"Data out of range\"\n-222,\"Data out of range\"\n-222,\"Data out of range\"\n-222,\"Data out of range\"\n-222,\"Data out of range\"\n-222,\"Data out of range\"\n-222,\"Data out of range\"\n-222,\"Data out of range\"\n-222,\"Data out of range\"\n-222,\"Data out of range\"\n-222,\"Data out of range\"\n-222,\"Data out of range\"\n-222,\"Data out of range\"\n-222,\"Data out of range\"\n-222,\"Data out of range\"\n-222,\"Data out of range\"\n-222,\"Data out of range\"\n-222,\"Data out of range\"\n-222,\"Data out of range\"\n-222,\"Data out of range\"\n-222,\"Data out of range\"\n-222,\"Data out of range\"\n-222,\"Data out of range\"\n-222,\"Data out of range\"\n-222,\"Data out of range\"\n-222,\"Data out of range\"\n-222,\"Data out of range\"\n-222,\"Data out of range\"\n-222,\"Data out of range\"\n-222,\"Data out of range\"\n-222,\"Data out of range\"\n-222,\"Data out of range\"\n-222,\"Data out of range\"\n-222,\"Data out of range\"\n-222,\"Data out of range\"\n-222,\"Data out of range\"\n-222,\"Data out of range\"\n-222,\"Data out of range\"\n-222,\"Data out of range\"\n-222,\"Data out of range\"\n-222,\"Data out of range\"\n-222,\"Data out of range\"\n-222,\"Data out of range\"\n-222,\"Data out of range\"\n-222,\"Data out of range\"\n-222,\"Data out of range\"\n-222,\"Data out of range\"\n-222,\"Data out of range\"\n-222,\"Data out of range\"\n-222,\"Data out of range\"\n-222,\"Data out of range\"\n-222,\"Data out of range\"\n-222,\"Data out of range\"\n-222,\"Data out of range\"\n-222,\"Data out of range\"\n-222,\"Data out of range\"\n-222,\"Data out of range\"\n-222,\"Data out of range\"\n-222,\"Data out of range\"\n-222,\"Data out of range\"\n-222,\"Data out of range\"\n-222,\"Data out of range\"\n-222,\"Data out of range\"\n-222,\"Data out of range\"\n-222,\"Data out of range\"\n-222,\"Data out of range\"\n-222,\"Data out of range\"\n-222,\"Data out of range\"\n-222,\"Data out of range\"\n-222,\"Data out of range\"\n-222,\"Data out of range\"\n-222,\"Data out of range\"\n-222,\"Data out of range\"\n-222,\"Data out of range\"\n-222,\"Data out of range\"\n-222,\"Data out of range\"\n-222,\"Data out of range\"\n-222,\"Data out of range\"\n-222,\"Data out of range\"\n-222,\"Data out of range\"\n-222,\"Data out of range\"\n-222,\"Data out of range\"\n-222,\"Data out of range\"\n-222,\"Data out of range\"\n-222,\"Data out of range\"\n-222,\"Data out of range\"\n-222,\"Data out of range\"\n-222,\"Data out of range\"\n-222,\"Data out of range\"\n-222,\"Data out of range\"\n-222,\"Data out of range\"\n-222,\"Data out of range\"\n-222,\"Data out of range\"\n-222,\"Data out of range\"\n-222,\"Data out of range\"\n-222,\"Data out of range\"\n-222,\"Data out of range\"\n-222,\"Data out of range\"\n-222,\"Data out of range\"\n-222,\"Data out of range\"\n-222,\"Data out of range\"\n-222,\"Data out of range\"\n-222,\"Data out of range\"\n-222,\"Data out of range\"\n-222,\"Data out of range\"\n-222,\"Data out of range\"\n-222,\"Data out of range\"\n-222,\"Data out of range\"\n-222,\"Data out of range\"\n-222,\"Data out of range\"\n-222,\"Data out of range\"\n-222,\"Data out of range\"\n-222,\"Data out of range\"\n-222,\"Data out of range\"\n-222,\"Data out of range\"\n-222,\"Data out of range\"\n-222,\"Data out of range\"\n-222,\"Data out of range\"\n-222,\"Data out of range\"\n-222,\"Data out of range\"\n-222,\"Data out of range\"\n-222,\"Data out of range\"\n-222,\"Data out of range\"\n-222,\"Data out of range\"\n-222,\"Data out of range\"\n-222,\"Data out of range\"\n-222,\"Data out of range\"\n-222,\"Data out of range\"\n-222,\"Data out of range\"\n-222,\"Data out of range\"\n-222,\"Data out of range\"\n-222,\"Data out of range\"\n-222,\"Data out of range\"\n-222,\"Data out of range\"\n-222,\"Data out of range\"\n-222,\"Data out of range\"\n-222,\"Data out of range\"\n-222,\"Data out of range\"\n-222,\"Data out of range\"\n-222,\"Data out of range\"\n-222,\"Data out of range\"\n-222,\"Data out of range\"\n-222,\"Data out of range\"\n-222,\"Data out of range\"\n-222,\"Data out of range\"\n-222,\"Data out of range\"\n-222,\"Data out of range\"\n-222,\"Data out of range\"\n-222,\"Data out of range\"\n-222,\"Data out of range\"\n-222,\"Data out of range\"\n-222,\"Data out of range\"\n-222,\"Data out of range\"\n-222,\"Data out of range\"\n-222,\"Data out of range\"\n-222,\"Data out of range\"\n-222,\"Data out of range\"\n-222,\"Data out of range\"\n-222,\"Data out of range\"\n-222,\"Data out of range\"\n-222,\"Data out of range\"\n-222,\"Data out of range\"\n-222,\"Data out of range\"\n-222,\"Data out of range\"\n-222,\"Data out of range\"\n-222,\"Data out of range\"\n-222,\"Data out of range\"\n-222,\"Data out of range\"\n-222,\"Data out of range\"\n-222,\"Data out of range\"\n-222,\"Data out of range\"\n-222,\"Data out of range\"\n-222,\"Data out of range\"\n-222,\"Data out of range\"\n-222,\"Data out of range\"\n-222,\"Data out of range\"\n-222,\"Data out of range\"\n-222,\"Data out of range\"\n-222,\"Data out of range\"\n-222,\"Data out of range\"\n-222,\"Data out of range\"\n-222,\"Data out of range\"\n-222,\"Data out of range\"\n-222,\"Data out of range\"\n-222,\"Data out of range\"\n-222,\"Data out of range\"\n-222,\"Data out of range\"\n-222,\"Data out of range\"\n-222,\"Data out of range\"\n-222,\"Data out of range\"\n-222,\"Data out of range\"\n-222,\"Data out of range\"\n-222,\"Data out of range\"\n-222,\"Data out of range\"\n-222,\"Data out of range\"\n-222,\"Data out of range\"\n-222,\"Data out of range\"\n-222,\"Data out of range\"\n-222,\"Data out of range\"\n-222,\"Data out of range\"\n-222,\"Data out of range\"\n-222,\"Data out of range\"\n-222,\"Data out of range\"\n-222,\"Data out of range\"\n-222,\"Data out of range\"\n-222,\"Data out of range\"\n-222,\"Data out of range\"\n-222,\"Data out of range\"\n-222,\"Data out of range\"\n-222,\"Data out of range\"\n-222,\"Data out of range\"\n-222,\"Data out of range\"\n-222,\"Data out of range\"\n-222,\"Data out of range\"\n-222,\"Data out of range\"\n-222,\"Data out of range\"\n-222,\"Data out of range\"\n-222,\"Data out of range\"\n-222,\"Data out of range\"\n-222,\"Data out of range\"\n-222,\"Data out of range\"\n-222,\"Data out of range\"\n-222,\"Data out of range\"\n-222,\"Data out of range\"\n-222,\"Data out of range\"\n-222,\"Data out of range\"\n-222,\"Data out of range\"\n-222,\"Data out of range\"\n-222,\"Data out of range\"\n-222,\"Data out of range\"\n-222,\"Data out of range\"\n-222,\"Data out of range\"\n-222,\"Data out of range\"\n-222,\"Data out of range\"\n-222,\"Data out of range\"\n-222,\"Data out of range\"\n-222,\"Data out of range\"\n-222,\"Data out of range\"\n-222,\"Data out of range\"\n-222,\"Data out of range\"\n-222,\"Data out of range\"\n-222,\"Data out of range\"\n-222,\"Data out of range\"\n-222,\"Data out of range\"\n-222,\"Data out of range\"\n-222,\"Data out of range\"\n-222,\"Data out of range\"\n-222,\"Data out of range\"\n-222,\"Data out of range\"\n-222,\"Data out of range\"\n-222,\"Data out of range\"\n-222,\"Data out of range\"\n-222,\"Data out of range\"\n-222,\"Data out of range\"\n-222,\"Data out of range\"\n-222,\"Data out of range\"\n-222,\"Data out of range\"\n-222,\"Data out of range\"\n-222,\"Data out of range\"\n-222,\"Data out of range\"\n-222,\"Data out of range\"\n-222,\"Data out of range\"\n-222,\"Data out of range\"\n-222,\"Data out of range\"\n-222,\"Data out of range\"\n-222,\"Data out of range\"\n-222,\"Data out of range\"\n-222,\"Data out of range\"\n-222,\"Data out of range\"\n-222,\"Data out of range\"\n-222,\"Data out of range\"\n-222,\"Data out of range\"\n-222,\"Data out of range\"\n-222,\"Data out of range\"\n-222,\"Data out of range\"\n-222,\"Data out of range\"\n-222,\"Data out of range\"\n-222,\"Data out of range\"\n-222,\"Data out of range\"\n-222,\"Data out of range\"\n-222,\"Data out of range\"\n-222,\"Data out of range\"\n-222,\"Data out of range\"\n-222,\"Data out of range\"\n-222,\"Data out of range\"\n-222,\"Data out of range\"\n-222,\"Data out of range\"\n-222,\"Data out of range\"\n-222,\"Data out of range\"\n-222,\"Data out of range\"\n-222,\"Data out of range\"\n-222,\"Data out of range\"\n-222,\"Data out of range\"\n-222,\"Data out of range\"\n-222,\"Data out of range\"\n-222,\"Data out of range\"\n-222,\"Data out of range\"\n-222,\"Data out of range\"\n-222,\"Data out of range\"\n-222,\"Data out of range\"\n-222,\"Data out of range\"\n-222,\"Data out of range\"\n-222,\"Data out of range\"\n-222,\"Data out of range\"\n-222,\"Data out of range\"\n-222,\"Data out of range\"\n-222,\"Data out of range\"\n-222,\"Data out of range\"\n-222,\"Data out of range\"\n-222,\"Data out of range\"\n-222,\"Data out of range\"\n-222,\"Data out of range\"\n-222,\"Data out of range\"\n-222,\"Data out of range\"\n-222,\"Data out of range\"\n-222,\"Data out of range\"\n-222,\"Data out of range\"\n-222,\"Data out of range\"\n-222,\"Data out of range\"\n-222,\"Data out of range\"\n-222,\"Data out of range\"\n-222,\"Data out of range\"\n-222,\"Data out of range\"\n-222,\"Data out of range\"\n-222,\"Data out of range\"\n-222,\"Data out of range\"\n-222,\"Data out of range\"\n-222,\"Data out of range\"\n-222,\"Data out of range\"\n-222,\"Data out of range\"\n-222,\"Data out of range\"\n-222,\"Data out of range\"\n-222,\"Data out of range\"\n-222,\"Data out of range\"\n-222,\"Data out of range\"\n-222,\"Data out of range\"\n-222,\"Data out of range\"\n-222,\"Data out of range\"\n-222,\"Data out of range\"\n-222,\"Data out of range\"\n-222,\"Data out of range\"\n-222,\"Data out of range\"\n-222,\"Data out of range\"\n-222,\"Data out of range\"\n-222,\"Data out of range\"\n-222,\"Data out of range\"\n-222,\"Data out of range\"\n-222,\"Data out of range\"\n-222,\"Data out of range\"\n-222,\"Data out of range\"\n-222,\"Data out of range\"\n-222,\"Data out of range\"\n-222,\"Data out of range\"\n-222,\"Data out of range\"\n-222,\"Data out of range\"\n-222,\"Data out of range\"\n-222,\"Data out of range\"\n-222,\"Data out of range\"\n-222,\"Data out of range\"\n-222,\"Data out of range\"\n-222,\"Data out of range\"\n-222,\"Data out of range\"\n-222,\"Data out of range\"\n-222,\"Data out of range\"\n-222,\"Data out of range\"\n-222,\"Data out of range\"\n-222,\"Data out of range\"\n-222,\"Data out of range\"\n-222,\"Data out of range\"\n-222,\"Data out of range\"\n-222,\"Data out of range\"\n-222,\"Data out of range\"\n-222,\"Data out of range\"\n-222,\"Data out of range\"\n-222,\"Data out of range\"\n-222,\"Data out of range\"\n-222,\"Data out of range\"\n-222,\"Data out of range\"\n-222,\"Data out of range\"\n-222,\"Data out of range\"\n-222,\"Data out of range\"\n-222,\"Data out of range\"\n-222,\"Data out of range\"\n-222,\"Data out of range\"\n-222,\"Data out of range\"\n-222,\"Data out of range\"\n-222,\"Data out of range\"\n-222,\"Data out of range\"\n-222,\"Data out of range\"\n-222,\"Data out of range\"\n-222,\"Data out of range\"\n-222,\"Data out of range\"\n-222,\"Data out of range\"\n-222,\"Data out of range\"\n-222,\"Data out of range\"\n-222,\"Data out of range\"\n-222,\"Data out of range\"\n-222,\"Data out of range\"\n-222,\"Data out of range\"\n-222,\"Data out of range\"\n-222,\"Data out of range\"\n-222,\"Data out of range\"\n-222,\"Data out of range\"\n-222,\"Data out of range\"\n-222,\"Data out of range\"\n-222,\"Data out of range\"\n-222,\"Data out of range\"\n-222,\"Data out of range\"\n-222,\"Data out of range\"\n-222,\"Data out of range\"\n-222,\"Data out of range\"\n-222,\"Data out of range\"\n-222,\"Data out of range\"\n-222,\"Data out of range\"\n-222,\"Data out of range\"\n-222,\"Data out of range\"\n-222,\"Data out of range\"\n-222,\"Data out of range\"\n-222,\"Data out of range\"\n-222,\"Data out of range\"\n-222,\"Data out of range\"\n-222,\"Data out of range\"\n-222,\"Data out of range\"\n-222,\"Data out of range\"\n-222,\"Data out of range\"\n-222,\"Data out of range\"\n-222,\"Data out of range\"\n-222,\"Data out of range\"\n-222,\"Data out of range\"\n-222,\"Data out of range\"\n-222,\"Data out of range\"\n-222,\"Data out of range\"\n-222,\"Data out of range\"\n-222,\"Data out of range\"\n-222,\"Data out of range\"\n-222,\"Data out of range\"\n-222,\"Data out of range\"\n-222,\"Data out of range\"\n-222,\"Data out of range\"\n-222,\"Data out of range\"\n-222,\"Data out of range\"\n-222,\"Data out of range\"\n-222,\"Data out of range\"\n-222,\"Data out of range\"\n-222,\"Data out of range\"\n-222,\"Data out of range\"\n-222,\"Data out of range\"\n-222,\"Data out of range\"\n-222,\"Data out of range\"\n-222,\"Data out of range\"\n-222,\"Data out of range\"\n-222,\"Data out of range\"\n-222,\"Data out of range\"\n-222,\"Data out of range\"\n-222,\"Data out of range\"\n-222,\"Data out of range\"\n-222,\"Data out of range\"\n-222,\"Data out of range\"\n-222,\"Data out of range\"\n-222,\"Data out of range\"\n-222,\"Data out of range\"\n-222,\"Data out of range\"\n-222,\"Data out of range\"\n-222,\"Data out of range\"\n-222,\"Data out of range\"\n-222,\"Data out of range\"\n-222,\"Data out of range\"\n-222,\"Data out of range\"\n-222,\"Data out of range\"\n-222,\"Data out of range\"\n-222,\"Data out of range\"\n-222,\"Data out of range\"\n-222,\"Data out of range\"\n-222,\"Data out of range\"\n-222,\"Data out of range\"\n-222,\"Data out of range\"\n-222,\"Data out of range\"\n-222,\"Data out of range\"\n-222,\"Data out of range\"\n-222,\"Data out of range\"\n-222,\"Data out of range\"\n-222,\"Data out of range\"\n-222,\"Data out of range\"\n-222,\"Data out of range\"\n-222,\"Data out of range\"\n-222,\"Data out of range\"\n-222,\"Data out of range\"\n-222,\"Data out of range\"\n-222,\"Data out of range\"\n-222,\"Data out of range\"\n-222,\"Data out of range\"\n-222,\"Data out of range\"\n-222,\"Data out of range\"\n-222,\"Data out of range\"\n-222,\"Data out of range\"\n-222,\"Data out of range\"\n-222,\"Data out of range\"\n-222,\"Data out of range\"\n-222,\"Data out of range\"\n-222,\"Data out of range\"\n-222,\"Data out of range\"\n-222,\"Data out of range\"\n-222,\"Data out of range\"\n-222,\"Data out of range\"\n-222,\"Data out of range\"\n-222,\"Data out of range\"\n-222,\"Data out of range\"\n-222,\"Data out of range\"\n-222,\"Data out of range\"\n-222,\"Data out of range\"\n-222,\"Data out of range\"\n-222,\"Data out of range\"\n-222,\"Data out of range\"\n-222,\"Data out of range\"\n-222,\"Data out of range\"\n-222,\"Data out of range\"\n-222,\"Data out of range\"\n-222,\"Data out of range\"\n-222,\"Data out of range\"\n-222,\"Data out of range\"\n-222,\"Data out of range\"\n-222,\"Data out of range\"\n-222,\"Data out of range\"\n-222,\"Data out of range\"\n-222,\"Data out of range\"\n-222,\"Data out of range\"\n-222,\"Data out of range\"\n-222,\"Data out of range\"\n-222,\"Data out of range\"\n-222,\"Data out of range\"\n-222,\"Data out of range\"\n-222,\"Data out of range\"\n-222,\"Data out of range\"\n-222,\"Data out of range\"\n-222,\"Data out of range\"\n-222,\"Data out of range\"\n-222,\"Data out of range\"\n-222,\"Data out of range\"\n-222,\"Data out of range\"\n-222,\"Data out of range\"\n-222,\"Data out of range\"\n-222,\"Data out of range\"\n-222,\"Data out of range\"\n-222,\"Data out of range\"\n-222,\"Data out of range\"\n-222,\"Data out of range\"\n-222,\"Data out of range\"\n-222,\"Data out of range\"\n-222,\"Data out of range\"\n-222,\"Data out of range\"\n-222,\"Data out of range\"\n-222,\"Data out of range\"\n-222,\"Data out of range\"\n-222,\"Data out of range\"\n-222,\"Data out of range\"\n-222,\"Data out of range\"\n-222,\"Data out of range\"\n-222,\"Data out of range\"\n-222,\"Data out of range\"\n-222,\"Data out of range\"\n-222,\"Data out of range\"\n-222,\"Data out of range\"\n-222,\"Data out of range\"\n-222,\"Data out of range\"\n-222,\"Data out of range\"\n-222,\"Data out of range\"\n-222,\"Data out of range\"\n-222,\"Data out of range\"\n-222,\"Data out of range\"\n-222,\"Data out of range\"\n-222,\"Data out of range\"\n-222,\"Data out of range\"\n-222,\"Data out of range\"\n-222,\"Data out of range\"\n-222,\"Data out of range\"\n-222,\"Data out of range\"\n-222,\"Data out of range\"\n-222,\"Data out of range\"\n-222,\"Data out of range\"\n-222,\"Data out of range\"\n-222,\"Data out of range\"\n-222,\"Data out of range\"\n-222,\"Data out of range\"\n-222,\"Data out of range\"\n-222,\"Data out of range\"\n-222,\"Data out of range\"\n-222,\"Data out of range\"\n-222,\"Data out of range\"\n-222,\"Data out of range\"\n-222,\"Data out of range\"\n-222,\"Data out of range\"\n-222,\"Data out of range\"\n-222,\"Data out of range\"\n-222,\"Data out of range\"\n-222,\"Data out of range\"\n-222,\"Data out of range\"\n-222,\"Data out of range\"\n-222,\"Data out of range\"\n-222,\"Data out of range\"\n-222,\"Data out of range\"\n-222,\"Data out of range\"\n-222,\"Data out of range\"\n-222,\"Data out of range\"\n-222,\"Data out of range\"\n-222,\"Data out of range\"\n-222,\"Data out of range\"\n-222,\"Data out of range\"\n-222,\"Data out of range\"\n-222,\"Data out of range\"\n-222,\"Data out of range\"\n-222,\"Data out of range\"\n-222,\"Data out of range\"\n-222,\"Data out of range\"\n-222,\"Data out of range\"\n-222,\"Data out of range\"\n-222,\"Data out of range\"\n-222,\"Data out of range\"\n-222,\"Data out of range\"\n-222,\"Data out of range\"\n-222,\"Data out of range\"\n-222,\"Data out of range\"\n-222,\"Data out of range\"\n-222,\"Data out of range\"\n-222,\"Data out of range\"\n-222,\"Data out of range\"\n-222,\"Data out of range\"\n-222,\"Data out of range\"\n-222,\"Data out of range\"\n-222,\"Data out of range\"\n-222,\"Data out of range\"\n-222,\"Data out of range\"\n-222,\"Data out of range\"\n-222,\"Data out of range\"\n-222,\"Data out of range\"\n-222,\"Data out of range\"\n-222,\"Data out of range\"\n-222,\"Data out of range\"\n-222,\"Data out of range\"\n-222,\"Data out of range\"\n-222,\"Data out of range\"\n-222,\"Data out of range\"\n-222,\"Data out of range\"\n-222,\"Data out of range\"\n-222,\"Data out of range\"\n-222,\"Data out of range\"\n-222,\"Data out of range\"\n-222,\"Data out of range\"\n-222,\"Data out of range\"\n-222,\"Data out of range\"\n-222,\"Data out of range\"\n-222,\"Data out of range\"\n-222,\"Data out of range\"\n-222,\"Data out of range\"\n-222,\"Data out of range\"\n-222,\"Data out of range\"\n-222,\"Data out of range\"\n-222,\"Data out of range\"\n-222,\"Data out of range\"\n-222,\"Data out of range\"\n-222,\"Data out of range\"\n-222,\"Data out of range\"\n-222,\"Data out of range\"\n-222,\"Data out of range\"\n-222,\"Data out of range\"\n-222,\"Data out of range\"\n-222,\"Data out of range\"\n-222,\"Data out of range\"\n-222,\"Data out of range\"\n-222,\"Data out of range\"\n-222,\"Data out of range\"\n-222,\"Data out of range\"\n-222,\"Data out of range\"\n-222,\"Data out of range\"\n-222,\"Data out of range\"\n-222,\"Data out of range\"\n-222,\"Data out of range\"\n-222,\"Data out of range\"\n-222,\"Data out of range\"\n-222,\"Data out of range\"\n-222,\"Data out of range\"\n-222,\"Data out of range\"\n-222,\"Data out of range\"\n-222,\"Data out of range\"\n-222,\"Data out of range\"\n-222,\"Data out of range\"\n-222,\"Data out of range\"\n-222,\"Data out of range\"\n-222,\"Data out of range\"\n-222,\"Data out of range\"\n-222,\"Data out of range\"\n-222,\"Data out of range\"\n-222,\"Data out of range\"\n-222,\"Data out of range\"\n-222,\"Data out of range\"\n-222,\"Data out of range\"\n-222,\"Data out of range\"\n-222,\"Data out of range\"\n-222,\"Data out of range\"\n-222,\"Data out of range\"\n-222,\"Data out of range\"\n-222,\"Data out of range\"\n-222,\"Data out of range\"\n-222,\"Data out of range\"\n-222,\"Data out of range\"\n-222,\"Data out of range\"\n-222,\"Data out of range\"\n-222,\"Data out of range\"\n-222,\"Data out of range\"\n-222,\"Data out of range\"\n-222,\"Data out of range\"\n-222,\"Data out of range\"\n-222,\"Data out of range\"\n-222,\"Data out of range\"\n-222,\"Data out of range\"\n-222,\"Data out of range\"\n-222,\"Data out of range\"\n-222,\"Data out of range\"\n-222,\"Data out of range\"\n-222,\"Data out of range\"\n-222,\"Data out of range\"\n-222,\"Data out of range\"\n-222,\"Data out of range\"\n-222,\"Data out of range\"\n-222,\"Data out of range\"\n-222,\"Data out of range\"\n-222,\"Data out of range\"\n-222,\"Data out of range\"\n-222,\"Data out of range\"\n-222,\"Data out of range\"\n-222,\"Data out of range\"\n-222,\"Data out of range\"\n-222,\"Data out of range\"\n-222,\"Data out of range\"\n-222,\"Data out of range\"\n-222,\"Data out of range\"\n-222,\"Data out of range\"\n-222,\"Data out of range\"\n-222,\"Data out of range\"\n-222,\"Data out of range\"\n-222,\"Data out of range\"\n-222,\"Data out of range\"\n-222,\"Data out of range\"\n-222,\"Data out of range\"\n-222,\"Data out of range\"\n-222,\"Data out of range\"\n-222,\"Data out of range\"\n-222,\"Data out of range\"\n-222,\"Data out of range\"\n-222,\"Data out of range\"\n-222,\"Data out of range\"\n-222,\"Data out of range\"\n-222,\"Data out of range\"\n-222,\"Data out of range\"\n-222,\"Data out of range\"\n-222,\"Data out of range\"\n-222,\"Data out of range\"\n-222,\"Data out of range\"\n-222,\"Data out of range\"\n-222,\"Data out of range\"\n-222,\"Data out of range\"\n-222,\"Data out of range\"\n-222,\"Data out of range\"\n-222,\"Data out of range\"\n-222,\"Data out of range\"\n-222,\"Data out of range\"\n-222,\"Data out of range\"\n-222,\"Data out of range\"\n-222,\"Data out of range\"\n-222,\"Data out of range\"\n-222,\"Data out of range\"\n-222,\"Data out of range\"\n-222,\"Data out of range\"\n-222,\"Data out of range\"\n-222,\"Data out of range\"\n-222,\"Data out of range\"\n-222,\"Data out of range\"\n-222,\"Data out of range\"\n-222,\"Data out of range\"\n-222,\"Data out of range\"\n-222,\"Data out of range\"\n-222,\"Data out of range\"\n-222,\"Data out of range\"\n-222,\"Data out of range\"\n-222,\"Data out of range\"\n-222,\"Data out of range\"\n-222,\"Data out of range\"\n-222,\"Data out of range\"\n-222,\"Data out of range\"\n-222,\"Data out of range\"\n-222,\"Data out of range\"\n-222,\"Data out of range\"\n-222,\"Data out of range\"\n-222,\"Data out of range\"\n-222,\"Data out of range\"\n-222,\"Data out of range\"\n-222,\"Data out of range\"\n-222,\"Data out of range\"\n-222,\"Data out of range\"\n-222,\"Data out of range\"\n-222,\"Data out of range\"\n-222,\"Data out of range\"\n-222,\"Data out of range\"\n-222,\"Data out of range\"\n-222,\"Data out of range\"\n-222,\"Data out of range\"\n-222,\"Data out of range\"\n-222,\"Data out of range\"\n-222,\"Data out of range\"\n-222,\"Data out of range\"\n-222,\"Data out of range\"\n-222,\"Data out of range\"\n-222,\"Data out of range\"\n-222,\"Data out of range\"\n-222,\"Data out of range\"\n-222,\"Data out of range\"\n-222,\"Data out of range\"\n-222,\"Data out of range\"\n-222,\"Data out of range\"\n-222,\"Data out of range\"\n-222,\"Data out of range\"\n-222,\"Data out of range\"\n-222,\"Data out of range\"\n-222,\"Data out of range\"\n-222,\"Data out of range\"\n-222,\"Data out of range\"\n-222,\"Data out of range\"\n-222,\"Data out of range\"\n-222,\"Data out of range\"\n-222,\"Data out of range\"\n-222,\"Data out of range\"\n-222,\"Data out of range\"\n-222,\"Data out of range\"\n-222,\"Data out of range\"\n-222,\"Data out of range\"\n-222,\"Data out of range\"\n-222,\"Data out of range\"\n-222,\"Data out of range\"\n-222,\"Data out of range\"\n-222,\"Data out of range\"\n-222,\"Data out of range\"\n-222,\"Data out of range\"\n-222,\"Data out of range\"\n-222,\"Data out of range\"\n-222,\"Data out of range\"\n-222,\"Data out of range\"\n-222,\"Data out of range\"\n-222,\"Data out of range\"\n-222,\"Data out of range\"\n-222,\"Data out of range\"\n-222,\"Data out of range\"\n-222,\"Data out of range\"\n-222,\"Data out of range\"\n-222,\"Data out of range\"\n-222,\"Data out of range\"\n-222,\"Data out of range\"\n-222,\"Data out of range\"\n-222,\"Data out of range\"\n-222,\"Data out of range\"\n-222,\"Data out of range\"\n-222,\"Data out of range\"\n-222,\"Data out of range\"\n-222,\"Data out of range\"\n-222,\"Data out of range\"\n-222,\"Data out of range\"\n-222,\"Data out of range\"\n-222,\"Data out of range\"\n-222,\"Data out of range\"\n-222,\"Data out of range\"\n-222,\"Data out of range\"\n-222,\"Data out of range\"\n-222,\"Data out of range\"\n-222,\"Data out of range\"\n-222,\"Data out of range\"\n-222,\"Data out of range\"\n-222,\"Data out of range\"\n-222,\"Data out of range\"\n-222,\"Data out of range\"\n-222,\"Data out of range\"\n-222,\"Data out of range\"\n-222,\"Data out of range\"\n-222,\"Data out of range\"\n-222,\"Data out of range\"\n-222,\"Data out of range\"\n-222,\"Data out of range\"\n-222,\"Data out of range\"\n-222,\"Data out of range\"\n-222,\"Data out of range\"\n-222,\"Data out of range\"\n-222,\"Data out of range\"\n-222,\"Data out of range\"\n-222,\"Data out of range\"\n-222,\"Data out of range\"\n-222,\"Data out of range\"\n-222,\"Data out of range\"\n-222,\"Data out of range\"\n-222,\"Data out of range\"\n-222,\"Data out of range\"\n-222,\"Data out of range\"\n-222,\"Data out of range\"\n-222,\"Data out of range\"\n-222,\"Data out of range\"\n-222,\"Data out of range\"\n-222,\"Data out of range\"\n-222,\"Data out of range\"\n-222,\"Data out of range\"\n-222,\"Data out of range\"\n-222,\"Data out of range\"\n-222,\"Data out of range\"\n-222,\"Data out of range\"\n-222,\"Data out of range\"\n-222,\"Data out of range\"\n-222,\"Data out of range\"\n-222,\"Data out of range\"\n-222,\"Data out of range\"\n-222,\"Data out of range\"\n-222,\"Data out of range\"\n-222,\"Data out of range\"\n-222,\"Data out of range\"\n-222,\"Data out of range\"\n-222,\"Data out of range\"\n-222,\"Data out of range\"\n-222,\"Data out of range\"\n-222,\"Data out of range\"\n-222,\"Data out of range\"\n-222,\"Data out of range\"\n-222,\"Data out of range\"\n-222,\"Data out of range\"\n-222,\"Data out of range\"\n-222,\"Data out of range\"\n-222,\"Data out of range\"\n-222,\"Data out of range\"\n-222,\"Data out of range\"\n-222,\"Data out of range\"\n-222,\"Data out of range\"\n-222,\"Data out of range\"\n-222,\"Data out of range\"\n-222,\"Data out of range\"\n-222,\"Data out of range\"\n-222,\"Data out of range\"\n-222,\"Data out of range\"\n-222,\"Data out of range\"\n-222,\"Data out of range\"\n-222,\"Data out of range\"\n-222,\"Data out of range\"\n-222,\"Data out of range\"\n-222,\"Data out of range\"\n-222,\"Data out of range\"\n-222,\"Data out of range\"\n-222,\"Data out of range\"\n-222,\"Data out of range\"\n-222,\"Data out of range\"\n-222,\"Data out of range\"\n-222,\"Data out of range\"\n-222,\"Data out of range\"\n-222,\"Data out of range\"\n-222,\"Data out of range\"\n-222,\"Data out of range\"\n-222,\"Data out of range\"\n-222,\"Data out of range\"\n-222,\"Data out of range\"\n-222,\"Data out of range\"\n-222,\"Data out of range\"\n-222,\"Data out of range\"\n-222,\"Data out of range\"\n-222,\"Data out of range\"\n-222,\"Data out of range\"\n-222,\"Data out of range\"\n-222,\"Data out of range\"\n-222,\"Data out of range\"\n-222,\"Data out of range\"\n-222,\"Data out of range\"\n-222,\"Data out of range\"\n-222,\"Data out of range\"\n-222,\"Data out of range\"\n-222,\"Data out of range\"\n-222,\"Data out of range\"\n-222,\"Data out of range\"\n-222,\"Data out of range\"\n-222,\"Data out of range\"\n-222,\"Data out of range\"\n-222,\"Data out of range\"\n-222,\"Data out of range\"\n-222,\"Data out of range\"\n-222,\"Data out of range\"\n-222,\"Data out of range\"\n-222,\"Data out of range\"\n-222,\"Data out of range\"\n-222,\"Data out of range\"\n-222,\"Data out of range\"\n-222,\"Data out of range\"\n-222,\"Data out of range\"\n-222,\"Data out of range\"\n-222,\"Data out of range\"\n-222,\"Data out of range\"\n-222,\"Data out of range\"\n-222,\"Data out of range\"\n-222,\"Data out of range\"\n-222,\"Data out of range\"\n-222,\"Data out of range\"\n-222,\"Data out of range\"\n-222,\"Data out of range\"\n-222,\"Data out of range\"\n-222,\"Data out of range\"\n-222,\"Data out of range\"\n-222,\"Data out of range\"\n-222,\"Data out of range\"\n-222,\"Data out of range\"\n-222,\"Data out of range\"\n-222,\"Data out of range\"\n-222,\"Data out of range\"\n-222,\"Data out of range\"\n-222,\"Data out of range\"\n-222,\"Data out of range\"\n-222,\"Data out of range\"\n-222,\"Data out of range\"\n-222,\"Data out of range\"\n-222,\"Data out of range\"\n-222,\"Data out of range\"\n-222,\"Data out of range\"\n-222,\"Data out of range\"\n-222,\"Data out of range\"\n-222,\"Data out of range\"\n-222,\"Data out of range\"\n-222,\"Data out of range\"\n-222,\"Data out of range\"\n-222,\"Data out of range\"\n-222,\"Data out of range\"\n-222,\"Data out of range\"\n-222,\"Data out of range\"\n-222,\"Data out of range\"\n-222,\"Data out of range\"\n-222,\"Data out of range\"\n-222,\"Data out of range\"\n-222,\"Data out of range\"\n-222,\"Data out of range\"\n-222,\"Data out of range\"\n-222,\"Data out of range\"\n-222,\"Data out of range\"\n-222,\"Data out of range\"\n-222,\"Data out of range\"\n-222,\"Data out of range\"\n-222,\"Data out of range\"\n-222,\"Data out of range\"\n-222,\"Data out of range\"\n-222,\"Data out of range\"\n-222,\"Data out of range\"\n-222,\"Data out of range\"\n-222,\"Data out of range\"\n-222,\"Data out of range\"\n-222,\"Data out of range\"\n-222,\"Data out of range\"\n-222,\"Data out of range\"\n-222,\"Data out of range\"\n-222,\"Data out of range\"\n-222,\"Data out of range\"\n-222,\"Data out of range\"\n-222,\"Data out of range\"\n-222,\"Data out of range\"\n-222,\"Data out of range\"\n-222,\"Data out of range\"\n-222,\"Data out of range\"\n-222,\"Data out of range\"\n-222,\"Data out of range\"\n-222,\"Data out of range\"\n-222,\"Data out of range\"\n-222,\"Data out of range\"\n-222,\"Data out of range\"\n-222,\"Data out of range\"\n-222,\"Data out of range\"\n-222,\"Data out of range\"\n-222,\"Data out of range\"\n-222,\"Data out of range\"\n-222,\"Data out of range\"\n-222,\"Data out of range\"\n-222,\"Data out of range\"\n-222,\"Data out of range\"\n-222,\"Data out of range\"\n-222,\"Data out of range\"\n-222,\"Data out of range\"\n-222,\"Data out of range\"\n-222,\"Data out of range\"\n-222,\"Data out of range\"\n-222,\"Data out of range\"\n-222,\"Data out of range\"\n-222,\"Data out of range\"\n-222,\"Data out of range\"\n-222,\"Data out of range\"\n-222,\"Data out of range\"\n-222,\"Data out of range\"\n-222,\"Data out of range\"\n-222,\"Data out of range\"\n-222,\"Data out of range\"\n-222,\"Data out of range\"\n-222,\"Data out of range\"\n-222,\"Data out of range\"\n-222,\"Data out of range\"\n-222,\"Data out of range\"\n-222,\"Data out of range\"\n-222,\"Data out of range\"\n-222,\"Data out of range\"\n-222,\"Data out of range\"\n-222,\"Data out of range\"\n-222,\"Data out of range\"\n-222,\"Data out of range\"\n-222,\"Data out of range\"\n-222,\"Data out of range\"\n-222,\"Data out of range\"\n-222,\"Data out of range\"\n-222,\"Data out of range\"\n-222,\"Data out of range\"\n-222,\"Data out of range\"\n-222,\"Data out of range\"\n-222,\"Data out of range\"\n-222,\"Data out of range\"\n-222,\"Data out of range\"\n-222,\"Data out of range\"\n-222,\"Data out of range\"\n-222,\"Data out of range\"\n-222,\"Data out of range\"\n-222,\"Data out of range\"\n-222,\"Data out of range\"\n-222,\"Data out of range\"\n-222,\"Data out of range\"\n-222,\"Data out of range\"\n-222,\"Data out of range\"\n-222,\"Data out of range\"\n-222,\"Data out of range\"\n-222,\"Data out of range\"\n-222,\"Data out of range\"\n-222,\"Data out of range\"\n-222,\"Data out of range\"\n-222,\"Data out of range\"\n-222,\"Data out of range\"\n-222,\"Data out of range\"\n-222,\"Data out of range\"\n-222,\"Data out of range\"\n-222,\"Data out of range\"\n-222,\"Data out of range\"\n-222,\"Data out of range\"\n-222,\"Data out of range\"\n-222,\"Data out of range\"\n-222,\"Data out of range\"\n-222,\"Data out of range\"\n-222,\"Data out of range\"\n-222,\"Data out of range\"\n-222,\"Data out of range\"\n-222,\"Data out of range\"\n-222,\"Data out of range\"\n-222,\"Data out of range\"\n-222,\"Data out of range\"\n-222,\"Data out of range\"\n-222,\"Data out of range\"\n-222,\"Data out of range\"\n-222,\"Data out of range\"\n-222,\"Data out of range\"\n-222,\"Data out of range\"\n-222,\"Data out of range\"\n-222,\"Data out of range\"\n-222,\"Data out of range\"\n-222,\"Data out of range\"\n-222,\"Data out of range\"\n-222,\"Data out of range\"\n-222,\"Data out of range\"\n-222,\"Data out of range\"\n-222,\"Data out of range\"\n-222,\"Data out of range\"\n-222,\"Data out of range\"\n-222,\"Data out of range\"\n-222,\"Data out of range\"\n-222,\"Data out of range\"\n-222,\"Data out of range\"\n-222,\"Data out of range\"\n-222,\"Data out of range\"\n-222,\"Data out of range\"\n-222,\"Data out of range\"\n-222,\"Data out of range\"\n-222,\"Data out of range\"\n-222,\"Data out of range\"\n-222,\"Data out of range\"\n-222,\"Data out of range\"\n-222,\"Data out of range\"\n-222,\"Data out of range\"\n-222,\"Data out of range\"\n-222,\"Data out of range\"\n-222,\"Data out of range\"\n-222,\"Data out of range\"\n-222,\"Data out of range\"\n-222,\"Data out of range\"\n-222,\"Data out of range\"\n-222,\"Data out of range\"\n-222,\"Data out of range\"\n-222,\"Data out of range\"\n-222,\"Data out of range\"\n-222,\"Data out of range\"\n-222,\"Data out of range\"\n-222,\"Data out of range\"\n-222,\"Data out of range\"\n-222,\"Data out of range\"\n-222,\"Data out of range\"\n-222,\"Data out of range\"\n-222,\"Data out of range\"\n-222,\"Data out of range\"\n-222,\"Data out of range\"\n-222,\"Data out of range\"\n-222,\"Data out of range\"\n-222,\"Data out of range\"\n-222,\"Data out of range\"\n-222,\"Data out of range\"\n-222,\"Data out of range\"\n-222,\"Data out of range\"\n-222,\"Data out of range\"\n-222,\"Data out of range\"\n-222,\"Data out of range\"\n-222,\"Data out of range\"\n-222,\"Data out of range\"\n-222,\"Data out of range\"\n-222,\"Data out of range\"\n-222,\"Data out of range\"\n-222,\"Data out of range\"\n-222,\"Data out of range\"\n-222,\"Data out of range\"\n-222,\"Data out of range\"\n-222,\"Data out of range\"\n-222,\"Data out of range\"\n-222,\"Data out of range\"\n-222,\"Data out of range\"\n-222,\"Data out of range\"\n-222,\"Data out of range\"\n-222,\"Data out of range\"\n-222,\"Data out of range\"\n-222,\"Data out of range\"\n-222,\"Data out of range\"\n-222,\"Data out of range\"\n-222,\"Data out of range\"\n-222,\"Data out of range\"\n-222,\"Data out of range\"\n-222,\"Data out of range\"\n-222,\"Data out of range\"\n-222,\"Data out of range\"\n-222,\"Data out of range\"\n-222,\"Data out of range\"\n-222,\"Data out of range\"\n-222,\"Data out of range\"\n-222,\"Data out of range\"\n-222,\"Data out of range\"\n-222,\"Data out of range\"\n-222,\"Data out of range\"\n-222,\"Data out of range\"\n-222,\"Data out of range\"\n-222,\"Data out of range\"\n-222,\"Data out of range\"\n-222,\"Data out of range\"\n-222,\"Data out of range\"\n-222,\"Data out of range\"\n-222,\"Data out of range\"\n-222,\"Data out of range\"\n-222,\"Data out of range\"\n-222,\"Data out of range\"\n-222,\"Data out of range\"\n-222,\"Data out of range\"\n-222,\"Data out of range\"\n-222,\"Data out of range\"\n-222,\"Data out of range\"\n-222,\"Data out of range\"\n-222,\"Data out of range\"\n-222,\"Data out of range\"\n-222,\"Data out of range\"\n-222,\"Data out of range\"\n-222,\"Data out of range\"\n-222,\"Data out of range\"\n-222,\"Data out of range\"\n-222,\"Data out of range\"\n-222,\"Data out of range\"\n-222,\"Data out of range\"\n-222,\"Data out of range\"\n-222,\"Data out of range\"\n-222,\"Data out of range\"\n-222,\"Data out of range\"\n-222,\"Data out of range\"\n-222,\"Data out of range\"\n-222,\"Data out of range\"\n-222,\"Data out of range\"\n-222,\"Data out of range\"\n-222,\"Data out of range\"\n-222,\"Data out of range\"\n"
  out "AUTO?":bool
  out "Zero Value":dbl format="%#.3p"
  out "Rng":string
  in  "Range":i16=1 min=1 max=6 step=1
  in  "Mono Port":refnum<visa-resource-name>="COM10"
  out "IDN String":string="Thorlabs,PM100USB,P2000362,1.3.0\n"
  out "Sensor SN":string="10061433"
  out "Sensor Name":string="S120C"
  out "Reply":string=" 0.000 nm  ok\r\n" caption="Mono Response"
  # "Range Settings"
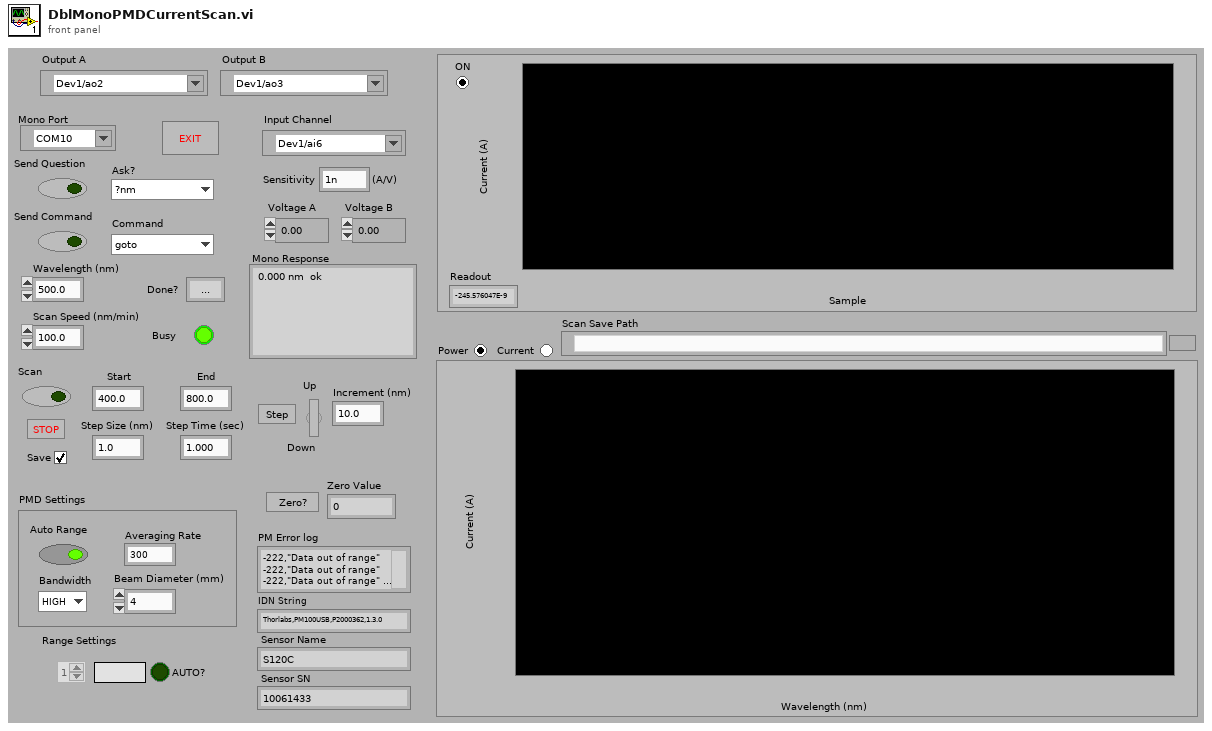
[diagram p1: front panel]
types:
  T1 = cluster{"Beam Diameter (mm)":dbl, "BWIn":u16, "Averaging Rate":i32, "Auto Range":bool}
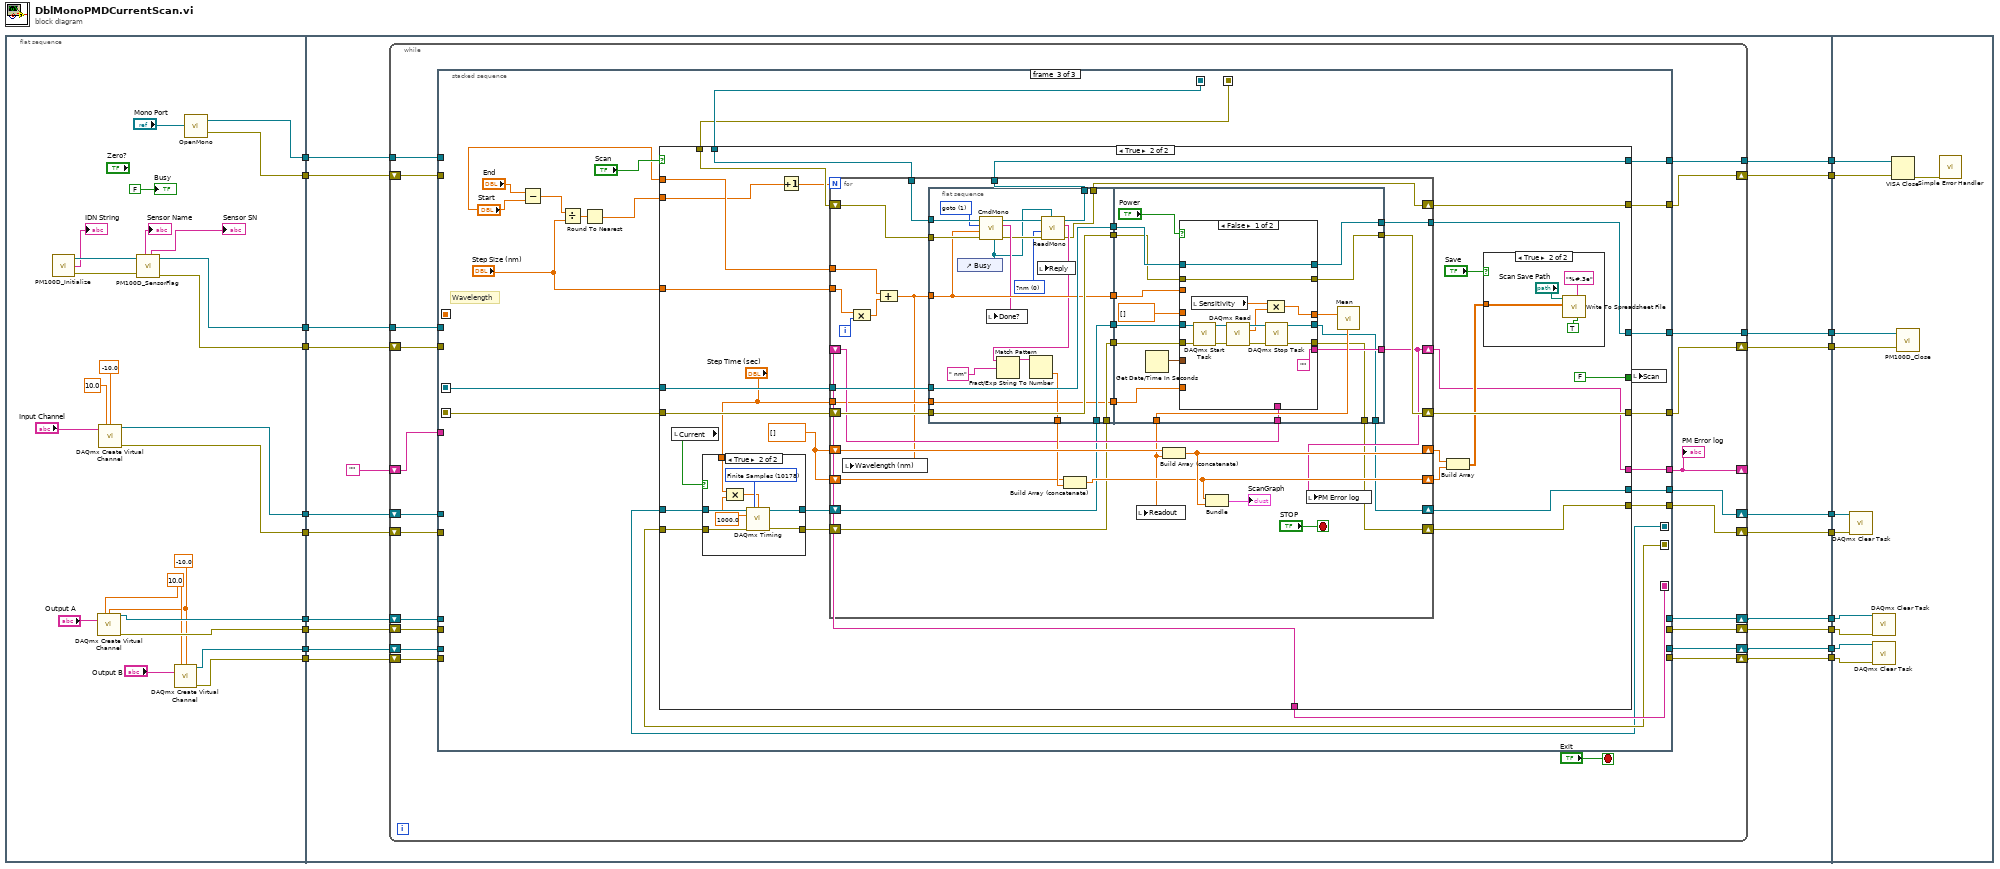
[diagram p0: block diagram]
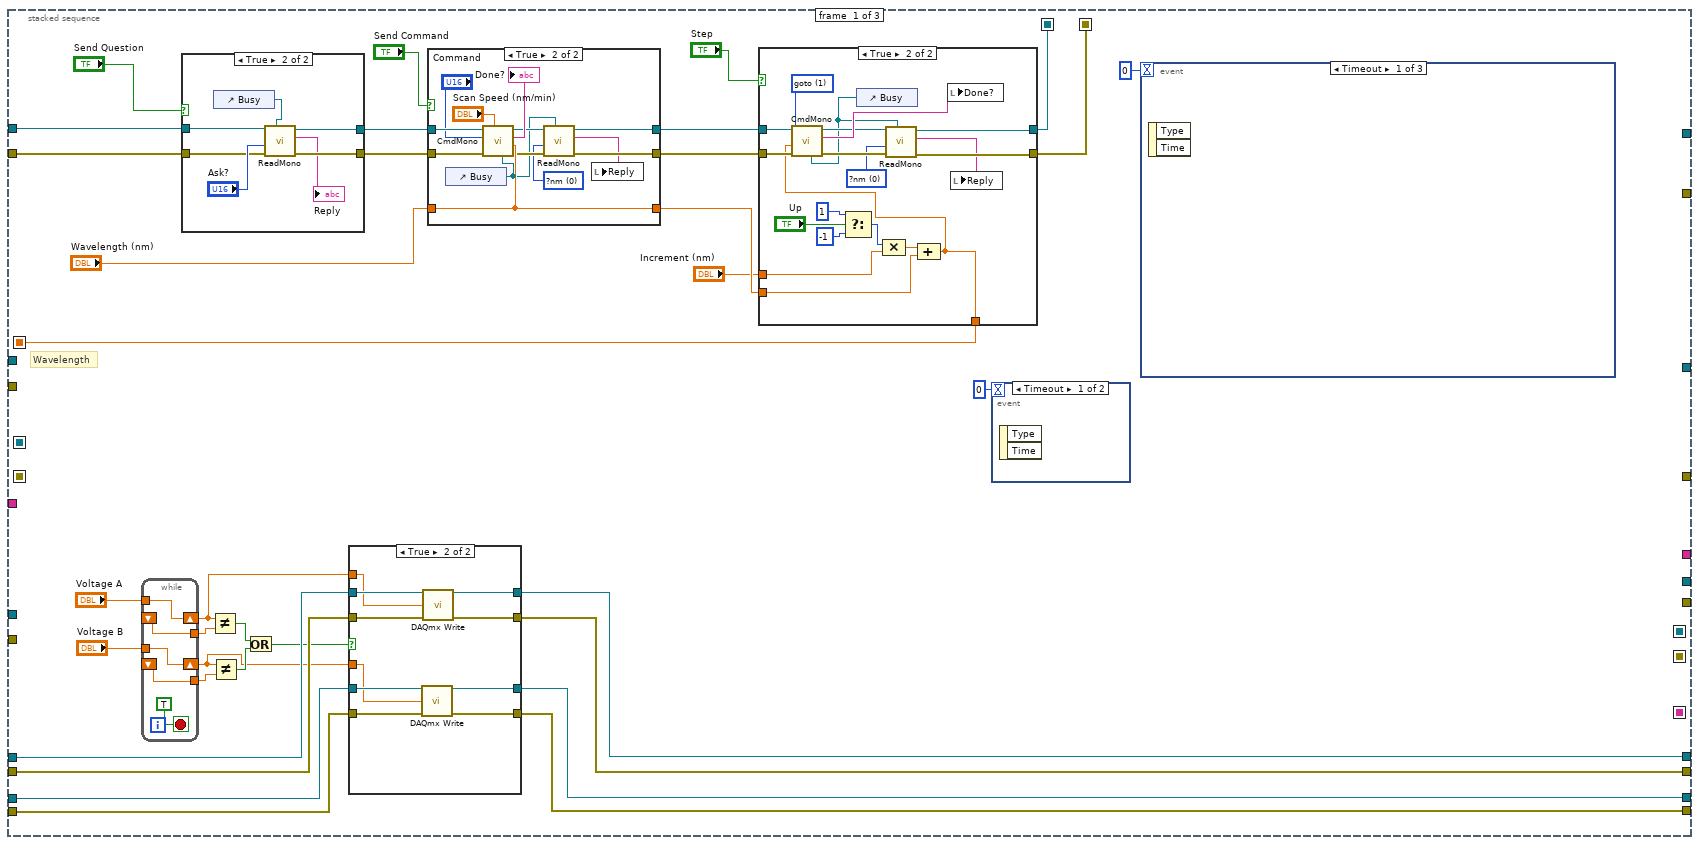
[diagram p2: hidden frame]
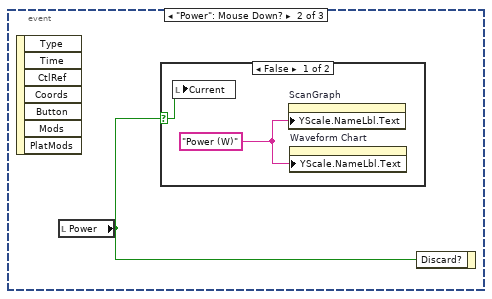
[diagram p4: hidden frame]
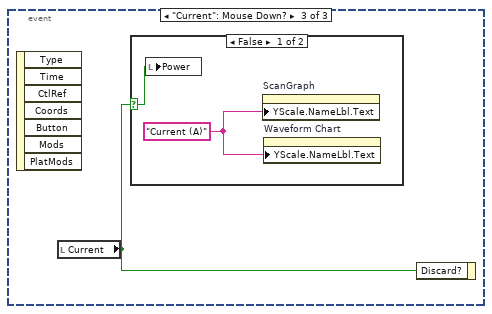
[diagram p6: hidden frame]
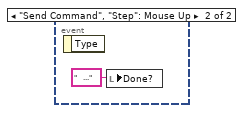
[diagram p8: hidden frame]
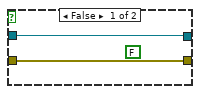
[diagram p11: hidden frame]
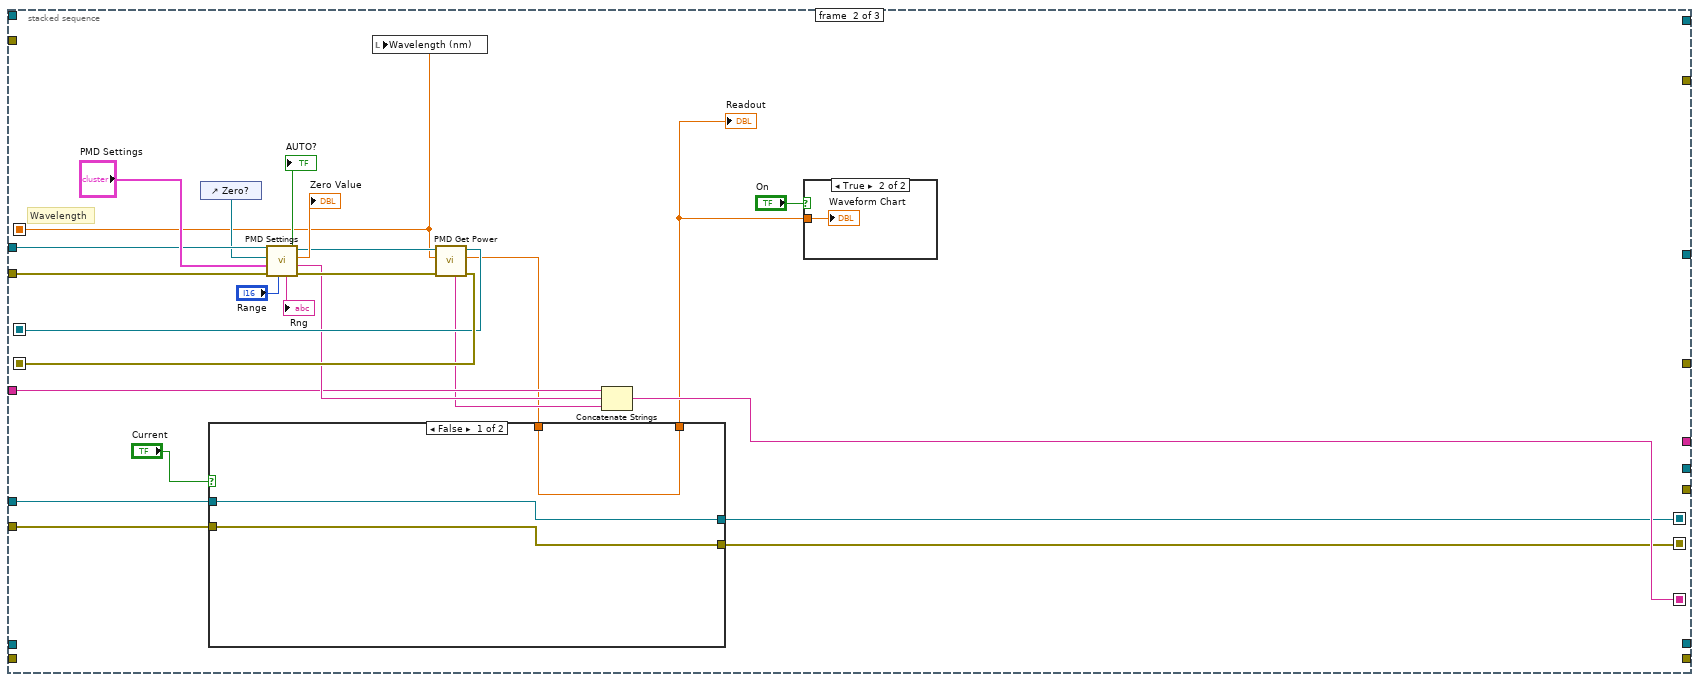
[diagram p12: hidden frame]
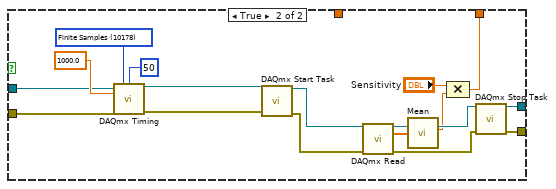
[diagram p13: hidden frame]
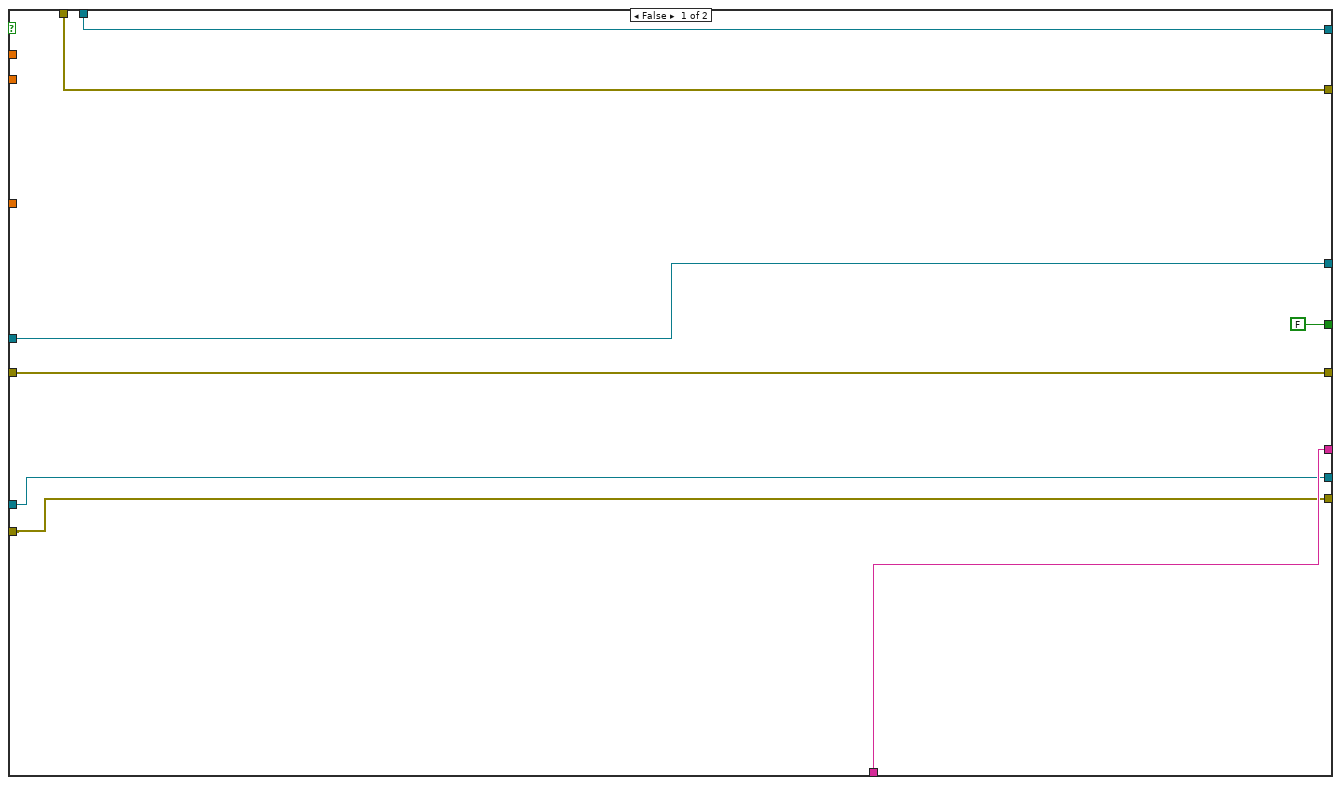
[diagram p15: hidden frame]
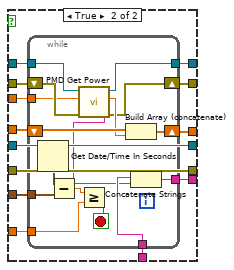
[diagram p18: hidden frame]
diagram:
  n1 = flat-sequence {
    tunnel: [w39] -> w20
    tunnel: [w38] -> w19
    tunnel: [w37] -> w18
    tunnel: [w36] -> w17
    tunnel: [w23] -> w12
    tunnel: [w24] -> w9
    tunnel: [w29] -> w8
    tunnel: [w30] -> w7
    tunnel: [w28] -> w6
    tunnel: [w27] -> w5
    tunnel: w20 -> [w64]
    tunnel: w19 -> [w65]
    tunnel: w18 -> [w63]
    tunnel: w17 -> [w62]
    tunnel: [w61] -> w16
    tunnel: [w60] -> w15
    tunnel: [w59] -> w14
    tunnel: [w58] -> w13
    tunnel: w12 -> [w55]
    tunnel: [w46] -> w11
    tunnel: [w45] -> w10
    tunnel: w9 -> [w56]
    tunnel: w8 -> [w54]
    tunnel: w7 -> [w53]
    tunnel: w6 -> [w52]
    tunnel: w5 -> [w51]
    tunnel: [w47] -> w4
    tunnel: [w48] -> w3
    tunnel: [w49] -> w2
    tunnel: [w50] -> w1
    tunnel: w16 -> [w437]
    tunnel: w15 -> [w436]
    tunnel: w14 -> [w435]
    tunnel: w13 -> [w434]
    tunnel: w11 -> [w432]
    tunnel: w10 -> [w433]
    tunnel: w4 -> [w431]
    tunnel: w3 -> [w430]
    tunnel: w2 -> [w429]
    tunnel: w1 -> [w428]
    frame #0 {
      w25 = -10.0 ("minimum value")
      w26 = 10.0 ("maximum value")
      n2 = call "PM100D_Initialize.vi"() -> ("error out"=w43:errorcluster, "Instrument"=→"IDN String":string, "VISA out"=w44:refnum<visa-resource-name>)  [unwired: 2 in, 1 out]
      n3 = call-poly <vilib>:"DAQmx Create Virtual Channel.vi"("maximum value"=w26, "minimum value"=w25, "physical channels"="Output A") -> ("task out"=w30:refnum<k21>, "error out"=w29:errorcluster)  [unwired: 11 in]
      n4 = call-poly <vilib>:"DAQmx Create Virtual Channel.vi"("maximum value"=10.0, "minimum value"=-10.0, "physical channels"="Input Channel") -> ("task out"=w24:refnum<k21>, "error out"=w23:errorcluster)  [unwired: 11 in]
      n5 = call "PM100D_SensorFlag.vi"("error in (no error)"=w43, "VISA in"=w44) -> ("error out"=w39:errorcluster, "VISA out"=w38:refnum<visa-resource-name>, "sn"=→"Sensor SN":string, "name"=→"Sensor Name":string)  [unwired: 2 in, 4 out]
      n6 = call-poly <vilib>:"DAQmx Create Virtual Channel.vi"("maximum value"=w26, "minimum value"=w25, "physical channels"="Output B") -> ("task out"=w27:refnum<k21>, "error out"=w28:errorcluster)  [unwired: 11 in]
      n7 = call "OpenMono.vi"("Mono Port"="Mono Port") -> ("VISA resource name out"=w37:refnum<visa-resource-name>, "error out"=w36:errorcluster)
      "Busy" <- FALSE ("Busy")
    }
    frame #1 {
      n8 = while {
        tunnel: w65 -> [w86]
        tunnel: w63 -> [w88]
        tunnel: [w83] -> w60
        tunnel: [w81] -> w58
        shift-right: [w80] -> w59
        shift-left: w64 -> [w85]
        shift-right: [w82] -> w61
        shift-left: w62 -> [w87]
        shift-right: [w78] -> _
        shift-left: "" -> [w79]
        shift-right: [w67] -> w45
        shift-left: w55 -> [w76]
        shift-right: [w66] -> w46
        shift-left: w56 -> [w77]
        shift-right: [w68] -> w50
        shift-left: w53 -> [w75]
        shift-right: [w69] -> w49
        shift-left: w54 -> [w74]
        shift-right: [w70] -> w48
        shift-left: w51 -> [w72]
        shift-right: [w71] -> w47
        shift-left: w52 -> [w73]
        stop <- "Exit" stop-if-true
        n9 = stacked-sequence {
          seq-local: [w107 _ _] -> [_ w203 _]
          seq-local: [w112 _ _] -> [_ _ w256]
          seq-local: [w111 _ _] -> [_ _ w255]
          seq-local: [_ w210 _] -> [_ _ w254]
          seq-local: [_ w211 _] -> [_ _ w253]
          seq-local: [_ w204 _] -> [_ _ w247]
          seq-local: [_ w198 _] -> [_ _ w243]
          seq-local: [_ w199 _] -> [_ _ w242]
          tunnel: w88 -> [w118 _ _]
          tunnel: w87 -> [w117 _ _]
          tunnel: w86 -> [_ w213 _]
          tunnel: w85 -> [_ w212 _]
          tunnel: [_ _ w252] -> w83
          tunnel: [_ _ w251] -> w82
          tunnel: [_ _ w250] -> w81
          tunnel: [_ _ w249] -> w80
          tunnel: w79 -> [_ w206 _]
          tunnel: [_ _ w246] -> w78
          tunnel: w77 -> [_ w197 _]
          tunnel: w76 -> [_ w196 _]
          tunnel: [_ _ w245] -> w66
          tunnel: [_ _ w244] -> w67
          tunnel: w75 -> [w102 _ _]
          tunnel: w74 -> [w103 _ _]
          tunnel: w73 -> [w105 _ _]
          tunnel: w72 -> [w104 _ _]
          tunnel: [w101 _ _] -> w71
          tunnel: [w100 _ _] -> w70
          tunnel: [w99 _ _] -> w69
          tunnel: [w98 _ _] -> w68
          frame #0 {
            # "Wavelength"
            n10 = while {
              shift-right: [w140] -> w89
              shift-left: _ -> [w139]
              tunnel: "Voltage B" -> [w140]
              tunnel: [w139] -> w94
              tunnel: "Voltage A" -> [w138]
              shift-right: [w138] -> w90
              shift-left: _ -> [w137]
              tunnel: [w137] -> w95
              stop <- TRUE stop-if-true
            }
            n11 = case shown="True" "Send Question" {
              tunnel: w118 -> [w188 w194]
              tunnel: w117 -> [w187 w193]
              tunnel: [w188 w192] -> w120
              tunnel: [w187 w191] -> w119
              frame False {
                (unwired) FALSE ("Read Error")
              }
              frame True {
                n12 = control-ref of="Busy"() -> (w189:refnum<vi>)
                n13 = call "ReadMono.vi"("Busy"=w189, "error in (no error)"=w193, "Cmd"="Ask?", "Mono Port"=w194) -> ("error out"=w191:errorcluster, "Response"=→"Reply":string, "Mono Port Out"=w192:refnum<visa-resource-name>)  [unwired: 2 in, 1 out]
              }
            }
            n14 = Not Equal?(x=w90, y=w95) -> (x != y?=w93:bool)
            n15 = Not Equal?(x=w89, y=w94) -> (x != y?=w92:bool)
            n16 = Or(x=w93, y=w92) -> (x .or. y?=w91:bool)
            n17 = case shown="True" w91 {
              tunnel: w105 -> [w123 w136]
              tunnel: w104 -> [w124 w135]
              tunnel: w103 -> [w125 w134]
              tunnel: w102 -> [w126 w133]
              tunnel: [w123 w132] -> w101
              tunnel: [w124 w131] -> w100
              tunnel: [w125 w130] -> w99
              tunnel: [w126 w129] -> w98
              tunnel: w90 -> [_ w127]
              tunnel: w89 -> [_ w128]
              frame False {
              }
              frame True {
                n18 = call-poly <vilib>:"DAQmx Write.vi"("task/channels in"=w135, "data"=w128, "error in"=w136) -> ("task out"=w131:refnum<k21>, "error out"=w132:errorcluster)  [unwired: 10 in, 1 out]
                n19 = call-poly <vilib>:"DAQmx Write.vi"("task/channels in"=w133, "data"=w127, "error in"=w134) -> ("task out"=w129:refnum<k21>, "error out"=w130:errorcluster)  [unwired: 10 in, 1 out]
              }
            }
            n20 = case shown="True" "Send Command" {
              tunnel: w120 -> [w173 w186]
              tunnel: w119 -> [w172 w185]
              tunnel: [w173 w178] -> w115
              tunnel: [w172 w177] -> w114
              tunnel: "Wavelength (nm)" -> [w171 w181]
              tunnel: [w171 w181] -> w113
              frame False {
              }
              frame True {
                w176 = u16 0 items=["?nm", "?nm/min", "?grating", "?turret", "?gratings"] ("Cmd")
                n21 = control-ref of="Busy"() -> (w174:refnum<vi>)
                n22 = call "CmdMono.vi"("Busy"=w174, "Scan Speed (nm/min)"="Scan Speed (nm/min)", "error in (no error)"=w185, "Wavelength (nm)"=w181, "Cmd"="Command", "Mono Port"=w186) -> ("error out"=w179:errorcluster, "Response"=→"Done?":string, "Mono Port Out"=w180:refnum<visa-resource-name>)  [unwired: 2 in, 1 out]
                n23 = call "ReadMono.vi"("Busy"=w174, "error in (no error)"=w179, "Cmd"=w176, "Mono Port"=w180) -> ("error out"=w177:errorcluster, "Response"=w175:string, "Mono Port Out"=w178:refnum<visa-resource-name>)  [unwired: 2 in, 1 out]
                n24 = local write "Reply"(w175) -> ()
              }
            }
            n25 = case shown="True" "Step" {
              tunnel: w115 -> [w151 w170]
              tunnel: w114 -> [w150 w169]
              tunnel: w113 -> [w149 w163]
              tunnel: [w151 w156] -> w112
              tunnel: [w150 w157] -> w111
              tunnel: "Increment (nm)" -> [_ w162]
              tunnel: [w149 w152] -> w107
              frame False {
              }
              frame True {
                w154 = u16 0 items=["?nm", "?nm/min", "?grating", "?turret", "?gratings"] ("Cmd")
                w161 = u16 1 items=["nm", "goto", "nm/min", "VIS grating", "IR grating"] ("Cmd")
                n26 = Select(t=1, s="Up", f=-1) -> (s? t:f=w168:i32)
                n27 = control-ref of="Busy"() -> (w153:refnum<vi>)
                n28 = Compound Arithmetic op=MULTIPLY(w168, w162) -> (w164:dbl)
                n29 = Compound Arithmetic op=ADD(w164, w163) -> (w152:dbl)
                n30 = call "CmdMono.vi"("Busy"=w153, "error in (no error)"=w169, "Wavelength (nm)"=w152, "Cmd"=w161, "Mono Port"=w170) -> ("error out"=w158:errorcluster, "Response"=w160:string, "Mono Port Out"=w159:refnum<visa-resource-name>)  [unwired: 3 in, 1 out]
                n31 = call "ReadMono.vi"("Busy"=w153, "error in (no error)"=w158, "Cmd"=w154, "Mono Port"=w159) -> ("error out"=w157:errorcluster, "Response"=w155:string, "Mono Port Out"=w156:refnum<visa-resource-name>)  [unwired: 2 in, 1 out]
                n32 = local write "Done?"(w160) -> ()
                n33 = local write "Reply"(w155) -> ()
              }
            }
            n34 = event shown="[0] Timeout" {
              selector: _ -> [_ _]
              dyn-events: _ -> [_ _]
              timeout: 0 -> [_ _]
              event Timeout {
                n35 = event-data() -> ()  [unwired: 1 in, 2 out]
              }
              event "Send Command", "Step": Mouse Up {
                n36 = event-data() -> ()  [unwired: 1 in, 1 out]
                n37 = local write "Done?"("   ..." ("Done?")) -> ()
              }
            }
            n38 = event shown="[0] Timeout" {
              selector: _ -> [_ _ _]
              dyn-events: _ -> [_ _ _]
              timeout: 0 -> [_ _ _]
              event Timeout {
                n39 = event-data() -> ()  [unwired: 1 in, 2 out]
              }
              event "Power": Mouse Down? {
                n40 = event-data() -> ()  [unwired: 1 in, 7 out]
                n41 = local read "Power"() -> (w142:bool)
                n42 = case shown="False" w142 {
                  selector: w142 -> [w144 _]
                  frame False {
                    w143 = "Power (W)" ("Y Scale.Name Label.Text")
                    n43 = local write "Current"(w144) -> ()
                    n44 = property on="ScanGraph" class="XYGraph (strict)"("YScale.NameLbl.Text"=w143) -> ()  [unwired: 2 in, 2 out]
                    n45 = property on="Waveform Chart" class="WFChart (strict)"("YScale.NameLbl.Text"=w143) -> ()  [unwired: 2 in, 2 out]
                  }
                  frame True {
                  }
                }
                n46 = event-data("Discard?"=w142) -> ()  [unwired: 1 in, 1 out]
              }
              event "Current": Mouse Down? {
                n47 = event-data() -> ()  [unwired: 1 in, 7 out]
                n48 = local read "Current"() -> (w145:bool)
                n49 = case shown="False" w145 {
                  selector: w145 -> [w146 _]
                  frame False {
                    w147 = "Current (A)" ("Y Scale.Name Label.Text")
                    n50 = local write "Power"(w146) -> ()
                    n51 = property on="ScanGraph" class="XYGraph (strict)"("YScale.NameLbl.Text"=w147) -> ()  [unwired: 2 in, 2 out]
                    n52 = property on="Waveform Chart" class="WFChart (strict)"("YScale.NameLbl.Text"=w147) -> ()  [unwired: 2 in, 2 out]
                  }
                  frame True {
                  }
                }
                n53 = event-data("Discard?"=w145) -> ()  [unwired: 1 in, 1 out]
              }
            }
          }
          frame #1 {
            # "Wavelength"
            n54 = control-ref of="Zero?"() -> (w208:refnum<vi>)
            n55 = call "PMD Settings.vi"("Visa In"=w213, "Zero?"=w208, "PMD Settings In"="PMD Settings", "Error In"=w212, "Range"="Range") -> ("AUTO?"=→"AUTO?":bool, "Rng"=→"Rng":string, "Visa Out"=w216:refnum<visa-resource-name>, "ZeroValue"=→"Zero Value":dbl, "PM Error log"=w207:string, "error out"=w215:errorcluster)
            n56 = local write "Wavelength (nm)"(w203) -> ()
            n57 = call "PMD Get Power.vi"("VISA In"=w216, "Wavelength (nm)"=w203, "error in"=w215) -> ("PMD Error"=w205:string, "VISA out"=w210:refnum<visa-resource-name>, "Readout value"=w202:dbl, "error out"=w211:errorcluster)  [unwired: 1 in, 2 out]
            n58 = case shown="False" "Current" {
              tunnel: w202 -> [w223 _]
              tunnel: w197 -> [w222 w226]
              tunnel: w196 -> [w221 w227]
              tunnel: [w223 w239] -> w200
              tunnel: [w221 w235] -> w198
              tunnel: [w222 w236] -> w199
              frame False {
              }
              frame True {
                w229 = 10178 items=["Finite Samples"=10178, "Continuous Samples"=10123, "Hardware Timed Single Point"=12522] ("sample mode")
                n59 = call-poly <vilib>:"DAQmx Timing.vi"("task/channels in"=w226, "sample mode"=w229, "samples per channel"=50, "rate"=1000.0, "error in"=w227) -> ("task out"=w225:refnum<k21>, "error out"=w224:errorcluster)  [unwired: 9 in]
                n60 = call <vilib>:"DAQmx Start Task.vi"("task/channels in"=w225, "error in"=w224) -> ("task out"=w237:refnum<k21>, "error out"=w238:errorcluster)  [unwired: 12 in]
                n61 = call-poly <vilib>:"DAQmx Read.vi"("task/channels in"=w237, "error in"=w238) -> ("task out"=w233:refnum<k21>, "data"=w232:dbl[], "error out"=w234:errorcluster)  [unwired: 11 in]
                n62 = call <vilib>:"Mean.vi"("X"=w232) -> ("mean"=w231:dbl)  [unwired: 1 out]
                n63 = Compound Arithmetic op=MULTIPLY("Sensitivity", w231) -> (w239:dbl)
                n64 = call <vilib>:"DAQmx Stop Task.vi"("task/channels in"=w233, "error in"=w234) -> ("task out"=w236:refnum<k21>, "error out"=w235:errorcluster)  [unwired: 12 in]
              }
            }
            "Readout" <- w200
            n65 = Concatenate Strings(w206, w207, w205) -> (w204:string)
            n66 = case shown="True" "On" {
              tunnel: w200 -> [_ w241]
              frame False {
              }
              frame True {
                "Waveform Chart" <- w241
              }
            }
          }
          frame #2 {
            # "Wavelength"
            n67 = Subtract(x="End", y="Start") -> (x-y=w261:dbl)
            n68 = Divide(x=w261, y="Step Size (nm)") -> (x/y=w260:dbl)
            n69 = Round To Nearest(number=w260) -> (nearest integer value=w259:dbl)
            n70 = case shown="True" "Scan" {
              tunnel: w259 -> [_ w294]
              tunnel: w255 -> [w269 w296]
              tunnel: w256 -> [w268 w297]
              tunnel: "Start" -> [_ w299]
              tunnel: "Step Size (nm)" -> [_ w298]
              tunnel: w254 -> [w271 w292]
              tunnel: w253 -> [w270 w291]
              tunnel: [w271 w280] -> w250
              tunnel: [w270 w290] -> w249
              tunnel: [w269 w289] -> w251
              tunnel: [w268 w288] -> w252
              tunnel: [FALSE ("Scan") FALSE ("Scan")] -> w248
              tunnel: w247 -> [w266 w282]
              tunnel: [w266 w281] -> w246
              tunnel: [w265 w279] -> w245
              tunnel: [w264 w278] -> w244
              tunnel: w243 -> [w264 w276]
              tunnel: w242 -> [w265 w275]
              frame False {
              }
              frame True {
                w295 = dbl[] []
                n71 = local read "Current"() -> (w277:bool)
                n72 = case shown="True" w277 {
                  tunnel: w276 -> [w300 w308]
                  tunnel: w275 -> [w301 w307]
                  tunnel: [w301 w306] -> w274
                  tunnel: [w300 w305] -> w273
                  tunnel: "Step Time (sec)" -> [_ w304]
                  frame False {
                  }
                  frame True {
                    w309 = 10178 items=["Finite Samples"=10178, "Continuous Samples"=10123, "Hardware Timed Single Point"=12522] ("sample mode")
                    w303 = 1000.0 ("rate")
                    n73 = Compound Arithmetic op=MULTIPLY(w304, w303) -> (w302:dbl)
                    n74 = call-poly <vilib>:"DAQmx Timing.vi"("task/channels in"=w307, "sample mode"=w309, "samples per channel"=w302, "rate"=w303, "error in"=w308) -> ("task out"=w306:refnum<k21>, "error out"=w305:errorcluster)  [unwired: 9 in]
                  }
                }
                n75 = Increment(x=w294) -> (x+1=w293:dbl)
                n76 = for {
                  N: w293 -> [_]
                  tunnel: w297 -> [w345]
                  tunnel: w299 -> [w341]
                  tunnel: w298 -> [w343]
                  shift-right: [w329] -> w287
                  shift-left: w295 -> [w347]
                  shift-right: [w340] -> w289
                  shift-left: w296 -> [w346]
                  shift-right: [w326] -> w286
                  shift-left: w295 -> [w327]
                  tunnel: w292 -> [w338]
                  shift-right: [w333] -> w290
                  shift-left: w291 -> [w337]
                  tunnel: [w332] -> w280
                  tunnel: [w331] -> w288
                  shift-right: [w324] -> w281
                  shift-left: w282 -> [w325]
                  shift-right: [w321] -> w278
                  shift-left: w273 -> [w316]
                  shift-right: [w320] -> w279
                  shift-left: w274 -> [w317]
                  tunnel: "Step Time (sec)" -> [w318]
                  i -> [w344]
                  stop <- "STOP" stop-if-true
                  n77 = Compound Arithmetic op=MULTIPLY(w343, w344) -> (w342:dbl)
                  n78 = Compound Arithmetic op=ADD(w341, w342) -> (w314:dbl)
                  n79 = local write "Wavelength (nm)"(w314) -> ()
                  n80 = flat-sequence {
                    tunnel: w346 -> [w367]
                    tunnel: w345 -> [w366]
                    tunnel: w314 -> [w362]
                    tunnel: [w351] -> w340
                    tunnel: w338 -> [w364]
                    tunnel: w337 -> [w363]
                    tunnel: [w364] -> w336
                    tunnel: [w363] -> w335
                    tunnel: [w362] -> w334
                    tunnel: [w356] -> w331
                    tunnel: [w352] -> w328
                    tunnel: w316 -> [w349]
                    tunnel: [w350] -> w323
                    tunnel: w317 -> [w350]
                    tunnel: [w349] -> w322
                    tunnel: [w348] -> w319
                    tunnel: w318 -> [w348]
                    tunnel: [w381] -> w315
                    tunnel: w336 -> [w380]
                    tunnel: w335 -> [w379]
                    tunnel: w334 -> [w378]
                    tunnel: [w374] -> w333
                    tunnel: [w377] -> w332
                    tunnel: w325 -> [w376]
                    tunnel: [w375] -> w324
                    tunnel: w323 -> [w372]
                    tunnel: w322 -> [w371]
                    tunnel: [w369] -> w320
                    tunnel: [w370] -> w321
                    tunnel: w319 -> [w373]
                    frame #0 {
                      w358 = u16 0 items=["?nm", "?nm/min", "?grating", "?turret", "?gratings"] ("Cmd")
                      w365 = u16 1 items=["nm", "goto", "nm/min", "VIS grating", "IR grating"] ("Cmd")
                      n81 = control-ref of="Busy"() -> (w357:refnum<vi>)
                      n82 = call "CmdMono.vi"("Busy"=w357, "error in (no error)"=w367, "Wavelength (nm)"=w362, "Cmd"=w365, "Mono Port"=w366) -> ("error out"=w359:errorcluster, "Response"=w361:string, "Mono Port Out"=w360:refnum<visa-resource-name>)  [unwired: 3 in, 1 out]
                      n83 = local write "Done?"(w361) -> ()
                      n84 = call "ReadMono.vi"("Busy"=w357, "error in (no error)"=w359, "Cmd"=w358, "Mono Port"=w360) -> ("error out"=w351:errorcluster, "Response"=w354:string, "Mono Port Out"=w356:refnum<visa-resource-name>)  [unwired: 2 in, 1 out]
                      n85 = Match Pattern(string=w354, regular expression=" nm") -> (before substring=w353:string)  [unwired: 1 in, 3 out]
                      n86 = Fract/Exp String To Number(string=w353) -> (number=w352:dbl)  [unwired: 3 in, 1 out]
                      n87 = local write "Reply"(w354) -> ()
                    }
                    frame #1 {
                      n88 = Get Date/Time In Seconds() -> (seconds since 1Jan1904=w383:timestamp)
                      n89 = case shown="False" "Power" {
                        tunnel: dbl[] [] -> [_ w411]
                        tunnel: w383 -> [_ w410]
                        tunnel: [w385 w409] -> w382
                        tunnel: w380 -> [w397 w408]
                        tunnel: w379 -> [w396 w407]
                        tunnel: w378 -> [_ w406]
                        tunnel: [w397 w405] -> w377
                        tunnel: w376 -> [_ w404]
                        tunnel: ["" w403] -> w375
                        tunnel: [w396 w402] -> w374
                        tunnel: w373 -> [_ w401]
                        tunnel: w372 -> [w395 w399]
                        tunnel: w371 -> [w394 w400]
                        tunnel: [w389 w400] -> w370
                        tunnel: [w388 w399] -> w369
                        frame False {
                          n90 = local read "Sensitivity"() -> (w386:dbl)
                          n91 = call <vilib>:"DAQmx Start Task.vi"("task/channels in"=w395, "error in"=w394) -> ("task out"=w393:refnum<k21>, "error out"=w392:errorcluster)  [unwired: 12 in]
                          n92 = call-poly <vilib>:"DAQmx Read.vi"("task/channels in"=w393, "error in"=w392) -> ("task out"=w391:refnum<k21>, "data"=w387:dbl[], "error out"=w390:errorcluster)  [unwired: 11 in]
                          n93 = call <vilib>:"DAQmx Stop Task.vi"("task/channels in"=w391, "error in"=w390) -> ("task out"=w388:refnum<k21>, "error out"=w389:errorcluster)  [unwired: 12 in]
                          n94 = Compound Arithmetic op=MULTIPLY(w386, w387) -> (w385:dbl[])
                        }
                        frame True {
                          n95 = while {
                            shift-right: [w426] -> w409
                            shift-left: w411 -> [w427]
                            tunnel: w410 -> [w424]
                            tunnel: w408 -> [w419]
                            tunnel: w406 -> [w415]
                            tunnel: [w417] -> w405
                            tunnel: w404 -> [w421]
                            tunnel: [w420] -> w403
                            shift-right: [w413] -> w402
                            shift-left: w407 -> [w418]
                            tunnel: w401 -> [w412]
                            stop <- w422 stop-if-true
                            n96 = Get Date/Time In Seconds() -> (seconds since 1Jan1904=w425:timestamp)
                            n97 = Subtract(x=w425, y=w424) -> (x-y=w423:dbl)
                            n98 = call "PMD Get Power.vi"("VISA In"=w419, "Wavelength (nm)"=w415, "error in"=w418) -> ("PMD Error"=w414:string, "VISA out"=w417:refnum<visa-resource-name>, "Readout value"=w416:dbl, "error out"=w413:errorcluster)  [unwired: 1 in, 2 out]
                            n99 = Greater Or Equal?(x=w423, y=w412) -> (x >= y?=w422:bool)
                            n100 = Build Array (concatenate)(w427, w416) -> (w426:dbl[])
                            n101 = Concatenate Strings(w421, w414) -> (w420:string)
                          }
                        }
                      }
                      n102 = call <vilib>:"Mean.vi"("X"=w382) -> ("mean"=w381:dbl)  [unwired: 1 out]
                    }
                  }
                  n103 = Build Array (concatenate)(w327, w328) -> (w326:dbl[])
                  n104 = local write "Readout"(w315) -> ()
                  n105 = Build Array (concatenate)(w347, w315) -> (w329:dbl[])
                  n106 = Bundle(w326, w329) -> (→"ScanGraph":cluster{dbl[], dbl[]})  [unwired: 1 in]
                  n107 = local write "PM Error log"(w324) -> ()
                }
                n108 = Build Array(w287, w286) -> (w285:dbl[][])
                n109 = case shown="True" "Save" {
                  tunnel: w285 -> [_ w310]
                  frame False {
                  }
                  frame True {
                    n110 = call-poly <vilib>:"Write To Spreadsheet File.vi"("transpose? (no:F)"=TRUE, "format (%.3f)"="%#.3e", "2D data"=w310, "file path (dialog if empty)"="Scan Save Path") -> ()  [unwired: 4 in, 1 out]
                  }
                }
              }
            }
            n111 = local write "Scan"(w248) -> ()
          }
        }
        "PM Error log" <- w78
      }
    }
    frame #2 {
      n112 = call <vilib>:"DAQmx Clear Task.vi"("task in"=w432, "error in"=w433) -> ()  [unwired: 13 in, 1 out]
      n113 = call <vilib>:"DAQmx Clear Task.vi"("task in"=w428, "error in"=w429) -> ()  [unwired: 13 in, 1 out]
      n114 = call <vilib>:"DAQmx Clear Task.vi"("task in"=w430, "error in"=w431) -> ()  [unwired: 13 in, 1 out]
      n115 = VISA Close(VISA resource name=w436, error in (no error)=w437) -> (error out=w438:errorcluster)
      n116 = call "PM100D_Close.vi"("error in (no error)"=w435, "VISA resource name"=w434) -> ()  [unwired: 2 in]
      n117 = call <vilib>:"Simple Error Handler.vi"("error in (no error)"=w438) -> ()  [unwired: 1 in, 8 out]
    }
  }
